vi "3.1.0_ECO_Mode.vi"(6 "Data in":T2, 8 "error in (no error)":errorcluster, 9 "AllControls In":T1, 10 "?":T3, 11 "Message Queue out":T4) -> (0 "error out":errorcluster, 1 "Flow":string, 2 "Data":T3, 3 "Message Queue Out":T4, 4 "Data out":T2)   [LabVIEW 2017]
uses:
  Depends/AMC/subVIs/TypeDefs/amc_Message Queue.ctl
  Depends/AMC/subVIs/TypeDefs/amc_Message.ctl
  Depends/Tools/Keyed Array/Tools_KeyedArray KeyedArray.ctl
  Ctrls/Data.ctl
  Ctrls/CSV_Data.ctl
  Ctrls/AllControls.ctl
  Ctrls/AlarmIndex.ctl
  DIPC 692 Daemon API/typdef/get_parameter.ctl
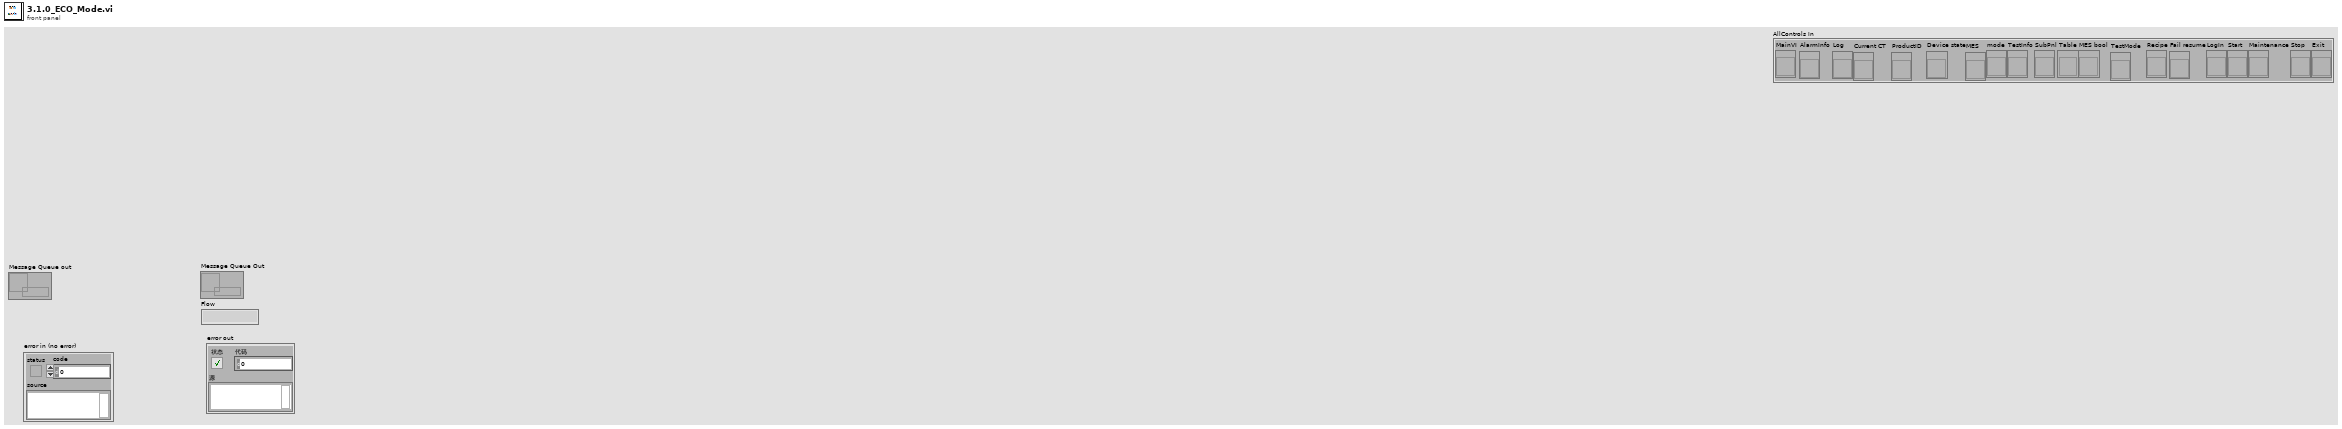
[diagram p1: front panel]
types:
  T1 = typedef "AllControls.ctl" = cluster{"MainVI":refnum<vi>, "AlarmInfo":refnum<vi>, "Log":refnum<vi>, "Current CT":refnum<vi>, "ProductID":refnum<vi>, "Device state":refnum<vi>, "MES":refnum<vi>, "mode":refnum<vi>, "TestInfo":refnum<vi>, "SubPnl":refnum<vi>, "Table":refnum<vi>, "MES bool":refnum<vi>, "TestMode":refnum<vi>, "Recipe":refnum<vi>, "Fail resume":refnum<vi>, "LogIn":refnum<vi>, "Start":refnum<vi>, "Maintenance":refnum<vi>, "Stop":refnum<vi>, "Exit":refnum<vi>}
  T2 = typedef "CSV_Data.ctl" = cluster{"Initialisation":cluster{"LMT - Connect UUT (con COM)":string, "LMT - Software Version (rrel)":string, "LMT - Write SKU file (wskuc)":string, "LMT - SKU file name":string, "Connect UUT DDM":string, "Read DDM EOL Timestamp - Mode":string, "Read DDM EOL Timestamp - Timestamp":string, "Read DDM EOL Timestamp - Rig ID":string, "Read DDM EOL Timestamp - Passmark ID":string, "Read DDM EOL Timestamp - Passmark Rev":string, "Software Version before flashing":string, "Read Hardware Serial":string, "UUT DDM SN":string, "Compare DDM SN with MES SN":string, "Backup PCBA Calibration EEPROM Response - CAL":string, "Flash Firmware Version":string, "Check SW Version":string, "Read DDM SW Version after flashing":string, "Set SKU Config":string, "Ready Status":string, "Set Device Mode to EOL":string, "DDM Parameter - Voltage":string, "DDM Parameter - Current":string, "DDM Parameter - Power":string, "DDM Parameter - Speed":string, "DDM Parameter - Pressure":string, "Tester Parameter - Voltage":string, "Tester Parameter - Current":string, "Tester Parameter - Power":string, "Tester Parameter - Ambient Pressure":string, "Tester Parameter - Ambient Temperature":string, "Calculated Parameter - DDM Pressure Corrected":string, "Calculated Parameter - DDM Real Power":string, "Calculated Parameter - Delta V":string}, "BEMF_Calibration":cluster{"Calibration Result - eol_cold_bemf_temp":string, "DDM Ambient Temp":string, "Restriction Plate Diameter":string, "Calibration Result - eol_bemf_mp_cold_coef_a":string, "Calibration Result - eol_bemf_mp_cold_coef_b":string, "Calibration Result - eol_bemf_mp_cold_coef_c":string, "Calibration Result - eol_bemf_lsi_cold_ref_coeffs":string, "Get - Calibration Result - eol_bemf_lsi_speed":string, "Get - Calibration Result - eol_bemf_lsi_integral_0":string, "Calibration Result - eol_bemf_lsi_integral_1":string, "Get - Calibration Result - eol_bemf_lsi_integral_2":string, "Get - Calibration Result - eol_cold_bemf":string, "Get - Calibration Result - eol_cold_bemf_fisf":string, "Finalise Calibration":string, "Compare -Calibration Result - eol_cold_bemf":string, "Compare -Calibration Result - eol_cold_bemf_fisf":string}, "ECO":cluster{"Reset Power Tune":string, "Reset BEMF FISF Calibration":string, "Restriction Plate Diameter":string, "ECO - Stabilisation Time":string, "ECO - DDM Parameter - Voltage":string, "ECO - DDM Parameter - Current":string, "ECO - DDM Parameter - Power":string, "ECO - DDM Parameter - Measured Power":string, "ECO - DDM Parameter - Speed":string, "ECO - DDM Parameter - Pressure":string, "ECO - Tester Parameter - Voltage":string, "ECO - Tester Parameter - Current":string, "ECO - Tester Parameter - Power":string, "ECO - Tester Parameter - Ambient Pressure":string, "ECO - Tester Parameter - Ambient Temperature":string, "ECO - Tester Parameter - Ambient Humidity":string, "ECO - Calculated Parameter - DDM Pressure Corrected":string, "ECO - Calculated Parameter - DDM Real Power":string, "ECO - Calculated Parameter - Delta V":string, "ECO - Calculated Parameter - Flowrate":string, "ECO - Calculated Parameter - Airwatt":string, "ECO - Formula":string, "PT ECO - Power Tune Mode Status":string}, "BOOST":cluster{"Restriction Plate Diameter":string, "BOOST - Stabilisation Time":string, "BOOST - DDM Parameter - Voltage":string, "BOOST - DDM Parameter - Current":string, "BOOST - DDM Parameter - Power":string, "BOOST - DDM Parameter - Measured Power":string, "BOOST - DDM Parameter - Speed":string, "BOOST - DDM Parameter - Pressure":string, "BOOST - Tester Parameter - Voltage":string, "BOOST - Tester Parameter - Current":string, "BOOST - Tester Parameter - Power":string, "BOOST - Tester Parameter - Ambient Pressure":string, "BOOST - Tester Parameter - Ambient Temperature":string, "BOOST - Tester Parameter - Ambient Humidity":string, "BOOST - Calculated Parameter - DDM Pressure Corrected":string, "BOOST - Calculated Parameter - DDM Real Power":string, "BOOST - Calculated Parameter - Delta V":string, "BOOST - Calculated Parameter - Flowrate":string, "BOOST - Calculated Parameter - Airwatt":string, "BOOST - Get AM Presence":string, "Air Muscle Turn Off Status":string, "BOOST - Air Muscle Calculated Parameter - Airwatt B":string, "BOOST - Air Muscle Calculate Airwatt Delta":string, "PT BOOST - Power Tune Mode Status":string, "Finalise Calibration":string, "ECO - Get AW Calibration value":string, "BOOST - Get AW Calibration value":string}, "MAX":cluster{"Restriction Plate Diameter":string, "MAX - Stabilisation Time":string, "Get Average Delta Tmag (LSIdelta_FISFdelta_LSItmag_FISFtmag_IIRtmag)":string, "Get Average Delta Tmag FISF":string, "MAX - DDM Parameter - Voltage":string, "MAX - DDM Parameter - Current":string, "MAX - DDM Parameter - Power":string, "MAX - DDM Parameter - Measured Power":string, "MAX - DDM Parameter - Speed":string, "MAX - DDM Parameter - Pressure":string, "MAX - Tester Parameter - Voltage":string, "MAX - Tester Parameter - Current":string, "MAX - Tester Parameter - Power":string, "MAX - Tester Parameter - Ambient Pressure":string, "MAX - Tester Parameter - Ambient Temperature":string, "MAX - Tester Parameter - Ambient Humidity":string, "MAX - Calculated Parameter - DDM Pressure Corrected":string, "MAX - Calculated Parameter - DDM Real Power":string, "MAX - Calculated Parameter - Delta V":string, "MAX - Calculated Parameter - Flowrate":string, "MAX - Calculated Parameter - Airwatt":string, "MAX_FISF_Check_Average_Delta_Tmag":string, "MAX - FISF - BEMF Finetune Result":string, "MAX tune - Delta P1":string, "MAX tune - Calculated Parameter - Airwatt":string, "Calculate Delta Airwatts - MAX finetune - Delta P2":string, "MAX finetune - DDM Parameter - Voltage":string, "MAX finetune - DDM Parameter - Current":string, "MAX finetune - DDM Parameter - Power":string, "MAX finetune - DDM Parameter - Measured Power":string, "MAX finetune - DDM Parameter - Speed":string, "MAX finetune - DDM Parameter - Pressure":string, "MAX finetune - Tester Parameter - Voltage":string, "MAX finetune - Tester Parameter - Current":string, "MAX finetune - Tester Parameter - Power":string, "MAX finetune - Tester Parameter - Ambient Pressure":string, "MAX finetune - Tester Parameter - Ambient Temperature":string, "MAX finetune - Tester Parameter - Ambient Humidity":string, "MAX finetune - Calculated Parameter - DDM Pressure Corrected":string, "MAX finetune - Calculated Parameter - DDM Real Power":string, "MAX finetune - Calculated Parameter - Delta V":string, "MAX finetune - Calculated Parameter - Flowrate":string, "MAX finetune - Calculated Parameter - Airwatt":string, "Check Derate Result":string, "Delta Tmag FISF":string, "Get Hot BEMF Result":string, "Calculate delta Pressure":string, "Finalise Calibration":string, "Calculate & Check Delta BEMF":string, "Delta P Airwatts Value":string}, "LL":cluster{"DDM Ambient Temp":string, "Restriction Plate Diameter":string, "LL - DDM Parameter - Voltage":string, "LL - DDM Parameter - Current":string, "LL - DDM Parameter - Power":string, "LL - DDM Parameter - Measured Power":string, "LL - DDM Parameter - Speed":string, "LL - DDM Parameter - Pressure":string, "LL - Tester Parameter - Voltage":string, "LL - Tester Parameter - Current":string, "LL - Tester Parameter - Power":string, "LL - DDM Real Power":string, "LL - Calibrate Task Detect LL":string}, "HL":cluster{"HL - DDM Parameter - Voltage":string, "HL - DDM Parameter - Current":string, "HL - DDM Parameter - Power":string, "HL - DDM Parameter - Measured Power":string, "HL - DDM Parameter - Speed":string, "HL - DDM Parameter - Pressure":string, "HL - Tester Parameter - Voltage":string, "HL - Tester Parameter - Current":string, "HL - Tester Parameter - Power":string, "HL - DDM Real Power":string, "HL - Calibrate Task Detect HL":string}, "LH":cluster{"Restriction Plate Diameter":string, "LH - DDM Parameter - Voltage":string, "LH - DDM Parameter - Current":string, "LH - DDM Parameter - Power":string, "LH - DDM Parameter - Measured Power":string, "LH - DDM Parameter - Speed":string, "LH - DDM Parameter - Pressure":string, "LH - Tester Parameter - Voltage":string, "LH - Tester Parameter - Current":string, "LH - Tester Parameter - Power":string, "LH - DDM Real Power":string, "LH - Calibrate Task Detect LH":string}, "HH":cluster{"HH - DDM Parameter - Voltage":string, "HH - DDM Parameter - Current":string, "HH - DDM Parameter - Power":string, "HH - DDM Parameter - Measured Power":string, "HH - DDM Parameter - Speed":string, "HH - DDM Parameter - Pressure":string, "HH - Tester Parameter - Voltage":string, "HH - Tester Parameter - Current":string, "HH - Tester Parameter - Power":string, "HH - DDM Real Power":string, "HH - Calibrate Task Detect HH":string}, "Inlet Blockage Calibration":cluster{"Inlet Blockage Calibration - DDM Parameter - Voltage":string, "Inlet Blockage Calibration - DDM Parameter - Current":string, "Inlet Blockage Calibration - DDM Parameter - Power":string, "Inlet Blockage Calibration - DDM Parameter - Measured Power":string, "Inlet Blockage Calibration - DDM Parameter - Speed":string, "Inlet Blockage Calibration - DDM Parameter - Pressure":string, "Inlet Blockage Calibration - Tester Parameter - Voltage":string, "Inlet Blockage Calibration - Tester Parameter - Current":string, "Inlet Blockage Calibration - Tester Parameter - Power":string, "Inlet Blockage Calibration - DDM Real Power":string, "Calibration Inlet Blockage_E":string, "Finalise Calibration":string, "Get Task Detect LL":string, "Get Task Detect HL":string, "Get Task Detect LH":string, "Get Task Detect HH":string, "Calibration Inlet Blockage":string, "Calibration eol cold bemf temp":string}, "GOOD":cluster{"GOOD UNIT - Clear EEPROM Error Log":string, "GOOD UNIT - Write Product Timestamp - Mode":string, "GOOD UNIT - Write Product Timestamp - Timestamp":string, "GOOD UNIT - Write Product Timestamp - Rig ID":string, "GOOD UNIT - Write Product Timestamp - Passmark ID":string, "GOOD UNIT - Write Product Timestamp - Passmark Rev":string, "GOOD UNIT - Set Device Mode to PROD":string, "GOOD UNIT - Backup PCBA Calibration EEPROM Response":string, "GOOD UNIT - Check Security Bit":string, "GOOD UNIT - Set Calibration Lock":string, "GOOD UNIT - Get_Calibration_Lock":string, "GOOD UNIT - Disconnect UUT":string}, "NG":cluster{"NG UNIT - Read NVM Error":string, "NG UNIT - Set Device Mode to FCT":string, "NG UNIT - Backup PCBA Calibration EEPROM Response - CAL":string, "NG UNIT - Backup PCBA Calibration EEPROM Response - ERROR":string, "NG UNIT - Backup PCBA Calibration EEPROM Response - USAGE":string, "NG UNIT - Disconnect UUT":string}, "SN":string, "Table":string[][], "Count":cluster{"Total":i32, "OK":i32, "NG":i32, "Yield":dbl}, "Start Time":timestamp, "daemon reference":refnum<k5>, "CT":dbl, "Config":string[][], "OK/NG":bool, "Station ID":string, "MES DDM SN":string, "MES PCBA SN":string, "Retest":string, "Variant":string, "Initialisation_Status":cluster{"LMT - Connect UUT (con COM)":string, "LMT - Software Version (rrel)":string, "LMT - Write SKU file (wskuc)":string, "LMT - SKU file name":string, "Connect UUT DDM":string, "Read DDM EOL Timestamp - Mode":string, "Read DDM EOL Timestamp - Timestamp":string, "Read DDM EOL Timestamp - Rig ID":string, "Read DDM EOL Timestamp - Passmark ID":string, "Read DDM EOL Timestamp - Passmark Rev":string, "Software Version before flashing":string, "Read Hardware Serial":string, "UUT DDM SN":string, "Compare DDM SN with MES SN":string, "Backup PCBA Calibration EEPROM Response - CAL":string, "Flash Firmware Version":string, "Check SW Version":string, "Read DDM SW Version after flashing":string, "Set SKU Config":string, "Ready Status":string, "Set Device Mode to EOL":string, "DDM Parameter - Voltage":string, "DDM Parameter - Current":string, "DDM Parameter - Power":string, "DDM Parameter - Speed":string, "DDM Parameter - Pressure":string, "Tester Parameter - Voltage":string, "Tester Parameter - Current":string, "Tester Parameter - Power":string, "Tester Parameter - Ambient Pressure":string, "Tester Parameter - Ambient Temperature":string, "Calculated Parameter - DDM Pressure Corrected":string, "Calculated Parameter - DDM Real Power":string, "Calculated Parameter - Delta V":string}, "BEMF_Calibration_Status":cluster{"Calibration Result - eol_cold_bemf_temp":string, "DDM Ambient Temp":string, "Restriction Plate Diameter":string, "Calibration Result - eol_bemf_mp_cold_coef_a":string, "Calibration Result - eol_bemf_mp_cold_coef_b":string, "Calibration Result - eol_bemf_mp_cold_coef_c":string, "Calibration Result - eol_bemf_lsi_cold_ref_coeffs":string, "Get - Calibration Result - eol_bemf_lsi_speed":string, "Get - Calibration Result - eol_bemf_lsi_integral_0":string, "Calibration Result - eol_bemf_lsi_integral_1":string, "Get - Calibration Result - eol_bemf_lsi_integral_2":string, "Get - Calibration Result - eol_cold_bemf":string, "Get - Calibration Result - eol_cold_bemf_fisf":string, "Finalise Calibration":string, "Compare -Calibration Result - eol_cold_bemf":string, "Compare -Calibration Result - eol_cold_bemf_fisf":string}, "ECO_Status":cluster{"Reset Power Tune":string, "Reset BEMF FISF Calibration":string, "Restriction Plate Diameter":string, "ECO - Stabilisation Time":string, "ECO - DDM Parameter - Voltage":string, "ECO - DDM Parameter - Current":string, "ECO - DDM Parameter - Power":string, "ECO - DDM Parameter - Measured Power":string, "ECO - DDM Parameter - Speed":string, "ECO - DDM Parameter - Pressure":string, "ECO - Tester Parameter - Voltage":string, "ECO - Tester Parameter - Current":string, "ECO - Tester Parameter - Power":string, "ECO - Tester Parameter - Ambient Pressure":string, "ECO - Tester Parameter - Ambient Temperature":string, "ECO - Tester Parameter - Ambient Humidity":string, "ECO - Calculated Parameter - DDM Pressure Corrected":string, "ECO - Calculated Parameter - DDM Real Power":string, "ECO - Calculated Parameter - Delta V":string, "ECO - Calculated Parameter - Flowrate":string, "ECO - Calculated Parameter - Airwatt":string, "ECO - Formula":string, "PT ECO - Power Tune Mode Status":string}, "BOOST_Status":cluster{"Restriction Plate Diameter":string, "BOOST - Stabilisation Time":string, "BOOST - DDM Parameter - Voltage":string, "BOOST - DDM Parameter - Current":string, "BOOST - DDM Parameter - Power":string, "BOOST - DDM Parameter - Measured Power":string, "BOOST - DDM Parameter - Speed":string, "BOOST - DDM Parameter - Pressure":string, "BOOST - Tester Parameter - Voltage":string, "BOOST - Tester Parameter - Current":string, "BOOST - Tester Parameter - Power":string, "BOOST - Tester Parameter - Ambient Pressure":string, "BOOST - Tester Parameter - Ambient Temperature":string, "BOOST - Tester Parameter - Ambient Humidity":string, "BOOST - Calculated Parameter - DDM Pressure Corrected":string, "BOOST - Calculated Parameter - DDM Real Power":string, "BOOST - Calculated Parameter - Delta V":string, "BOOST - Calculated Parameter - Flowrate":string, "BOOST - Calculated Parameter - Airwatt":string, "BOOST - Get AM Presence":string, "Air Muscle Turn Off Status":string, "BOOST - Air Muscle Calculated Parameter - Airwatt B":string, "BOOST - Air Muscle Calculate Airwatt Delta":string, "PT BOOST - Power Tune Mode Status":string, "Finalise Calibration":string, "ECO - Get AW Calibration value":string, "BOOST - Get AW Calibration value":string}, "MAX_Status":cluster{"Restriction Plate Diameter":string, "MAX - Stabilisation Time":string, "Get Average Delta Tmag (LSIdelta_FISFdelta_LSItmag_FISFtmag_IIRtmag)":string, "Get Average Delta Tmag FISF":string, "MAX - DDM Parameter - Voltage":string, "MAX - DDM Parameter - Current":string, "MAX - DDM Parameter - Power":string, "MAX - DDM Parameter - Measured Power":string, "MAX - DDM Parameter - Speed":string, "MAX - DDM Parameter - Pressure":string, "MAX - Tester Parameter - Voltage":string, "MAX - Tester Parameter - Current":string, "MAX - Tester Parameter - Power":string, "MAX - Tester Parameter - Ambient Pressure":string, "MAX - Tester Parameter - Ambient Temperature":string, "MAX - Tester Parameter - Ambient Humidity":string, "MAX - Calculated Parameter - DDM Pressure Corrected":string, "MAX - Calculated Parameter - DDM Real Power":string, "MAX - Calculated Parameter - Delta V":string, "MAX - Calculated Parameter - Flowrate":string, "MAX - Calculated Parameter - Airwatt":string, "MAX_FISF_Check_Average_Delta_Tmag":string, "MAX - FISF - BEMF Finetune Result":string, "MAX tune - Delta P1":string, "MAX tune - Calculated Parameter - Airwatt":string, "Calculate Delta Airwatts - MAX finetune - Delta P2":string, "MAX finetune - DDM Parameter - Voltage":string, "MAX finetune - DDM Parameter - Current":string, "MAX finetune - DDM Parameter - Power":string, "MAX finetune - DDM Parameter - Measured Power":string, "MAX finetune - DDM Parameter - Speed":string, "MAX finetune - DDM Parameter - Pressure":string, "MAX finetune - Tester Parameter - Voltage":string, "MAX finetune - Tester Parameter - Current":string, "MAX finetune - Tester Parameter - Power":string, "MAX finetune - Tester Parameter - Ambient Pressure":string, "MAX finetune - Tester Parameter - Ambient Temperature":string, "MAX finetune - Tester Parameter - Ambient Humidity":string, "MAX finetune - Calculated Parameter - DDM Pressure Corrected":string, "MAX finetune - Calculated Parameter - DDM Real Power":string, "MAX finetune - Calculated Parameter - Delta V":string, "MAX finetune - Calculated Parameter - Flowrate":string, "MAX finetune - Calculated Parameter - Airwatt":string, "Check Derate Result":string, "Delta Tmag FISF":string, "Get Hot BEMF Result":string, "Calculate delta Pressure":string, "Finalise Calibration":string, "Calculate & Check Delta BEMF":string, "Delta P Airwatts Value":string}, "LL_Status":cluster{"DDM Ambient Temp":string, "Restriction Plate Diameter":string, "LL - DDM Parameter - Voltage":string, "LL - DDM Parameter - Current":string, "LL - DDM Parameter - Power":string, "LL - DDM Parameter - Measured Power":string, "LL - DDM Parameter - Speed":string, "LL - DDM Parameter - Pressure":string, "LL - Tester Parameter - Voltage":string, "LL - Tester Parameter - Current":string, "LL - Tester Parameter - Power":string, "LL - DDM Real Power":string, "LL - Calibrate Task Detect LL":string}, "HL_Status":cluster{"HL - DDM Parameter - Voltage":string, "HL - DDM Parameter - Current":string, "HL - DDM Parameter - Power":string, "HL - DDM Parameter - Measured Power":string, "HL - DDM Parameter - Speed":string, "HL - DDM Parameter - Pressure":string, "HL - Tester Parameter - Voltage":string, "HL - Tester Parameter - Current":string, "HL - Tester Parameter - Power":string, "HL - DDM Real Power":string, "HL - Calibrate Task Detect HL":string}, "LH_Status":cluster{"Restriction Plate Diameter":string, "LH - DDM Parameter - Voltage":string, "LH - DDM Parameter - Current":string, "LH - DDM Parameter - Power":string, "LH - DDM Parameter - Measured Power":string, "LH - DDM Parameter - Speed":string, "LH - DDM Parameter - Pressure":string, "LH - Tester Parameter - Voltage":string, "LH - Tester Parameter - Current":string, "LH - Tester Parameter - Power":string, "LH - DDM Real Power":string, "LH - Calibrate Task Detect LH":string}, "HH_Status":cluster{"HH - DDM Parameter - Voltage":string, "HH - DDM Parameter - Current":string, "HH - DDM Parameter - Power":string, "HH - DDM Parameter - Measured Power":string, "HH - DDM Parameter - Speed":string, "HH - DDM Parameter - Pressure":string, "HH - Tester Parameter - Voltage":string, "HH - Tester Parameter - Current":string, "HH - Tester Parameter - Power":string, "HH - DDM Real Power":string, "HH - Calibrate Task Detect HH":string}, "Inlet Blockage Calibration_Status":cluster{"Inlet Blockage Calibration - DDM Parameter - Voltage":string, "Inlet Blockage Calibration - DDM Parameter - Current":string, "Inlet Blockage Calibration - DDM Parameter - Power":string, "Inlet Blockage Calibration - DDM Parameter - Measured Power":string, "Inlet Blockage Calibration - DDM Parameter - Speed":string, "Inlet Blockage Calibration - DDM Parameter - Pressure":string, "Inlet Blockage Calibration - Tester Parameter - Voltage":string, "Inlet Blockage Calibration - Tester Parameter - Current":string, "Inlet Blockage Calibration - Tester Parameter - Power":string, "Inlet Blockage Calibration - DDM Real Power":string, "Calibration Inlet Blockage_E":string, "Finalise Calibration":string, "Get Task Detect LL":string, "Get Task Detect HL":string, "Get Task Detect LH":string, "Get Task Detect HH":string, "Calibration Inlet Blockage":string, "Calibration eol cold bemf temp":string}, "GOOD_Status":cluster{"GOOD UNIT - Clear EEPROM Error Log":string, "GOOD UNIT - Write Product Timestamp - Mode":string, "GOOD UNIT - Write Product Timestamp - Timestamp":string, "GOOD UNIT - Write Product Timestamp - Rig ID":string, "GOOD UNIT - Write Product Timestamp - Passmark ID":string, "GOOD UNIT - Write Product Timestamp - Passmark Rev":string, "GOOD UNIT - Set Device Mode to PROD":string, "GOOD UNIT - Backup PCBA Calibration EEPROM Response":string, "GOOD UNIT - Check Security Bit":string, "GOOD UNIT - Set Calibration Lock":string, "GOOD UNIT - Get_Calibration_Lock":string, "GOOD UNIT - Disconnect UUT":string}, "NG_Status":cluster{"NG UNIT - Read NVM Error":string, "NG UNIT - Set Device Mode to FCT":string, "NG UNIT - Backup PCBA Calibration EEPROM Response - CAL":string, "NG UNIT - Backup PCBA Calibration EEPROM Response - ERROR":string, "NG UNIT - Backup PCBA Calibration EEPROM Response - USAGE":string, "NG UNIT - Disconnect UUT":string}, "SKU":string, "Plate_Diameter":string, "Alarm":string}
  T3 = typedef "Data.ctl" = cluster{"Initialisation":cluster{"DDM_Parameter":dbl[], "DDM_Parameter_status":bool[], "Get_Tester_Parameter":dbl[], "Get_Tester_Parameter_status":bool[], "Cal_Tester_Parameter":dbl[], "Cal_Tester_Parameter_status":bool[], "sw_version_before_status":bool, "sw_version_after_status":bool, "Set_SKU_Config_With_LMT_status":bool, "FCT_timestamp_status":bool, "LMT_Connect_to_UUT_status":bool}, "BEMF_Calibration":cluster{"Read_ambient_temperature":dbl, "Calibration_Vaule":dbl[], "Calibration_Vaule _B":dbl[], "Calibration_Vaule_status":bool[], "Calibration_Vaule_B_status":bool[]}, "ECO":cluster{"DDM_Parameter":dbl[], "DDM_Parameter_status":bool[], "Get_Tester_Parameter":dbl[], "Get_Tester_Parameter_status":bool[], "Cal_Tester_Parameter":dbl[], "Cal_Tester_Parameter_status":bool[], "DDM_Parameter_after_power_tune":dbl[], "Get_Tester_Parameter_after_power_tune":dbl[], "Cal_Tester_Parameter_after_power_tune":dbl[], "Cal_Tester_Parameter_after_power_tune_status":bool[], "Delta_P":dbl}, "BOOST":cluster{"DDM_Parameter":dbl[], "DDM_Parameter_status":bool[], "Get_Tester_Parameter":dbl[], "Get_Tester_Parameter_status":bool[], "Cal_Tester_Parameter":dbl[], "Cal_Tester_Parameter_status":bool[], "DDM_Parameter_after_power_tune":dbl[], "Get_Tester_Parameter_after_power_tune":dbl[], "Cal_Tester_Parameter_after_power_tune":dbl[], "Cal_Tester_Parameter_after_power_tune_status":bool[], "airwatts_am_off":dbl, "AW_Delta_(AM_on_and_off)":dbl, "AW_Delta_(AM_on_and_off)_Status":bool, "Delta_P":dbl}, "MAX":cluster{"Average_Tmag_Data":cluster{"LSI Delta in degC":dbl, "FISF Delta in degc":dbl, "LSI Tmag in degC":dbl, "Fisf Tmag in degC":dbl, "IIR Tmag in degC":dbl}, "DDM_Parameter":dbl[], "DDM_Parameter_status":bool[], "Get_Tester_Parameter":dbl[], "Get_Tester_Parameter_status":bool[], "Cal_Tester_Parameter":dbl[], "BEMF_Finetune":cluster{"eol_bemf_mp_cold_coef_c":dbl, "eol_cold_bemf_fisf_offset":dbl}, "AW_Tune":cluster{"delta_P1":dbl, "delta_P_Setting":dbl}, "DDM_Parameter_after_Airwatts_Tune":dbl[], "Get_Tester_Parameter_after_Airwatts_Tune":dbl[], "Cal_Tester_Parameter_after_Airwatts_Tune":dbl[], "DDM_Parameter_after_Airwatts_Finetune":dbl[], "Get_Tester_Parameter_after_Airwatts_Finetune":dbl[], "Cal_Tester_Parameter_after_Airwatts_Finetune":dbl[], "AW_Finetune":cluster{"delta_P2":dbl, "delta_P_Setting":dbl}, "Delta_Tmag_after_tune":cluster{"LSI Delta in degC":dbl, "FISF Delta in degc":dbl, "LSI Tmag in degC":dbl, "Fisf Tmag in degC":dbl, "IIR Tmag in degC":dbl}, "Hot Bemf in mV":dbl, "DDM_Pressure":dbl, "Delta_Pressure":dbl, " Cold Bemf in mV":dbl, " delta Bemf":dbl, " delta p":dbl, "Delta_Pressure_status":bool, " delta Bemf_status":bool, "LSI Delta in degC_status":bool, "FISF Delta in degc_status":bool, "Max_check_derate_status_status":bool, "Average_All_data":dbl[][], "Average_Tmag_Data_status":bool[], "Average_Tmag_Data_after_tune_status":bool[], "Cal_Tester_Parameter_status":bool[], "Cal_Tester_Parameter_status_after_Airwatts_Tune":bool[], "Cal_Tester_Parameter_status_after_Airwatts_FineTune":bool[]}, "Task_Detect_Calib":cluster{"LL":cluster{"DDM_Parameter":dbl[], "DDM_Parameter_status":bool[], "Get_Tester_Parameter":dbl[], "Get_Tester_Parameter_status":bool[], "Set_task_detect_A":dbl, "Set_task_detect_A_Status":bool}, "HL":cluster{"DDM_Parameter":dbl[], "DDM_Parameter_status":bool[], "Get_Tester_Parameter":dbl[], "Get_Tester_Parameter_status":bool[], "Set_task_detect_B":dbl, "Set_task_detect_B_Status":bool}, "LH":cluster{"DDM_Parameter":dbl[], "DDM_Parameter_status":bool[], "Get_Tester_Parameter":dbl[], "Get_Tester_Parameter_status":bool[], "Set_task_detect_C":dbl, "Set_task_detect_C_Status":bool}, "HH":cluster{"DDM_Parameter":dbl[], "DDM_Parameter_status":bool[], "Get_Tester_Parameter":dbl[], "Get_Tester_Parameter_status":bool[], "Set_task_detect_D":dbl, "Read_and_check_calibration_Status":bool[], "Set_task_detect_D_Status":bool}, "Get_eol_inlet_blockage_E":dbl, "Calib_vaule":cluster{"Get_task_detect_LL":dbl, "Get_task_detect_HL":dbl, "Get_task_detect_LH":dbl, "Get_task_detect_HH":dbl, "eol_inlet_blockage":dbl, "eol_code_bemf_temp":dbl}, "calibrated temp":dbl, "Inlet_Blockage_Calibration":cluster{"DDM_Parameter":dbl[], "DDM_Parameter_status":bool[], "Get_Tester_Parameter":dbl[], "Get_Tester_Parameter_status":bool[]}, "Get_eol_inlet_blockage_E_Status":bool}, "good":cluster{"Write_Product_TS":cluster{"TIMESTAMP":i64, "RIG_ID":i64, "PASSMARK_ID":i64, "PASSMARK_REV":i64}, "Read_Product_TS":cluster{"TIMESTAMP":i64, "RIG_ID":i64, "PASSMARK_ID":i64, "PASSMARK_REV":i64}, "Good_Check_Secuity_Bit_Stauts":bool}}
  T4 = typedef "amc_Message Queue.ctl" = refnum<queue>
  T5 = typedef "HD Config.ctl" = cluster{" PC":cluster{"PC Address":u8[], "PC Port":i32}, "FCO":cluster{"COM":refnum<visa-resource-name>, "Baudrate":u32}, "DC Power ":cluster{"COM":refnum<visa-resource-name>, "Baudrate":u32}, "PW3336":cluster{"COM":refnum<visa-resource-name>, "Baudrate":u32}, "Lefoo":cluster{"COM":refnum<visa-resource-name>, "Baudrate":u32}, "AI Model":cluster{"COM":refnum<visa-resource-name>, "Baudrate":u32}, "DIPC":cluster{"COM":refnum<visa-resource-name>}, "NFC":cluster{"IP Address":string, "Port":u16, "Retry":u16}, "Motor":cluster{"COM":refnum<visa-resource-name>, "Baudrate":u32}, "Fail_resume_mode":bool, "GRR":bool}
  T6 = typedef "AlarmIndex.ctl" = enum16{"E-Stop", "Safety light grid", "UUT Sealing Cylinder HomePoint", "UUT Sealing Cylinder WorkPoint", "Orifice fixed Cylinder L HomePoint", "Orifice fixed Cylinder L WorkPoint", "Orifice fixed Cylinder R HomePoint", "Orifice fixed Cylinder R WorkPoint", "UUT Cylinder HomePoint", "UUT Cylinder WorkPoint", "Carrier fixed Cylinder L HomePoint", "Carrier fixed Cylinder L WorkPoint", "Carrier fixed Cylinder R HomePoint", "Carrier fixed Cylinder R WorkPoint", "Probe Cylinder HomePoint", "Probe Cylinder WorkPoint", "Motor Error", "Test Error"}
  T7 = typedef "get_parameter.ctl" = string
  T8 = typedef "Position Config.ctl" = cluster{"OrificeSize_12.7":i32, "OrificeSize_13":i32, "OrificeSize_30":i32, "OrificeSize_16":i32}
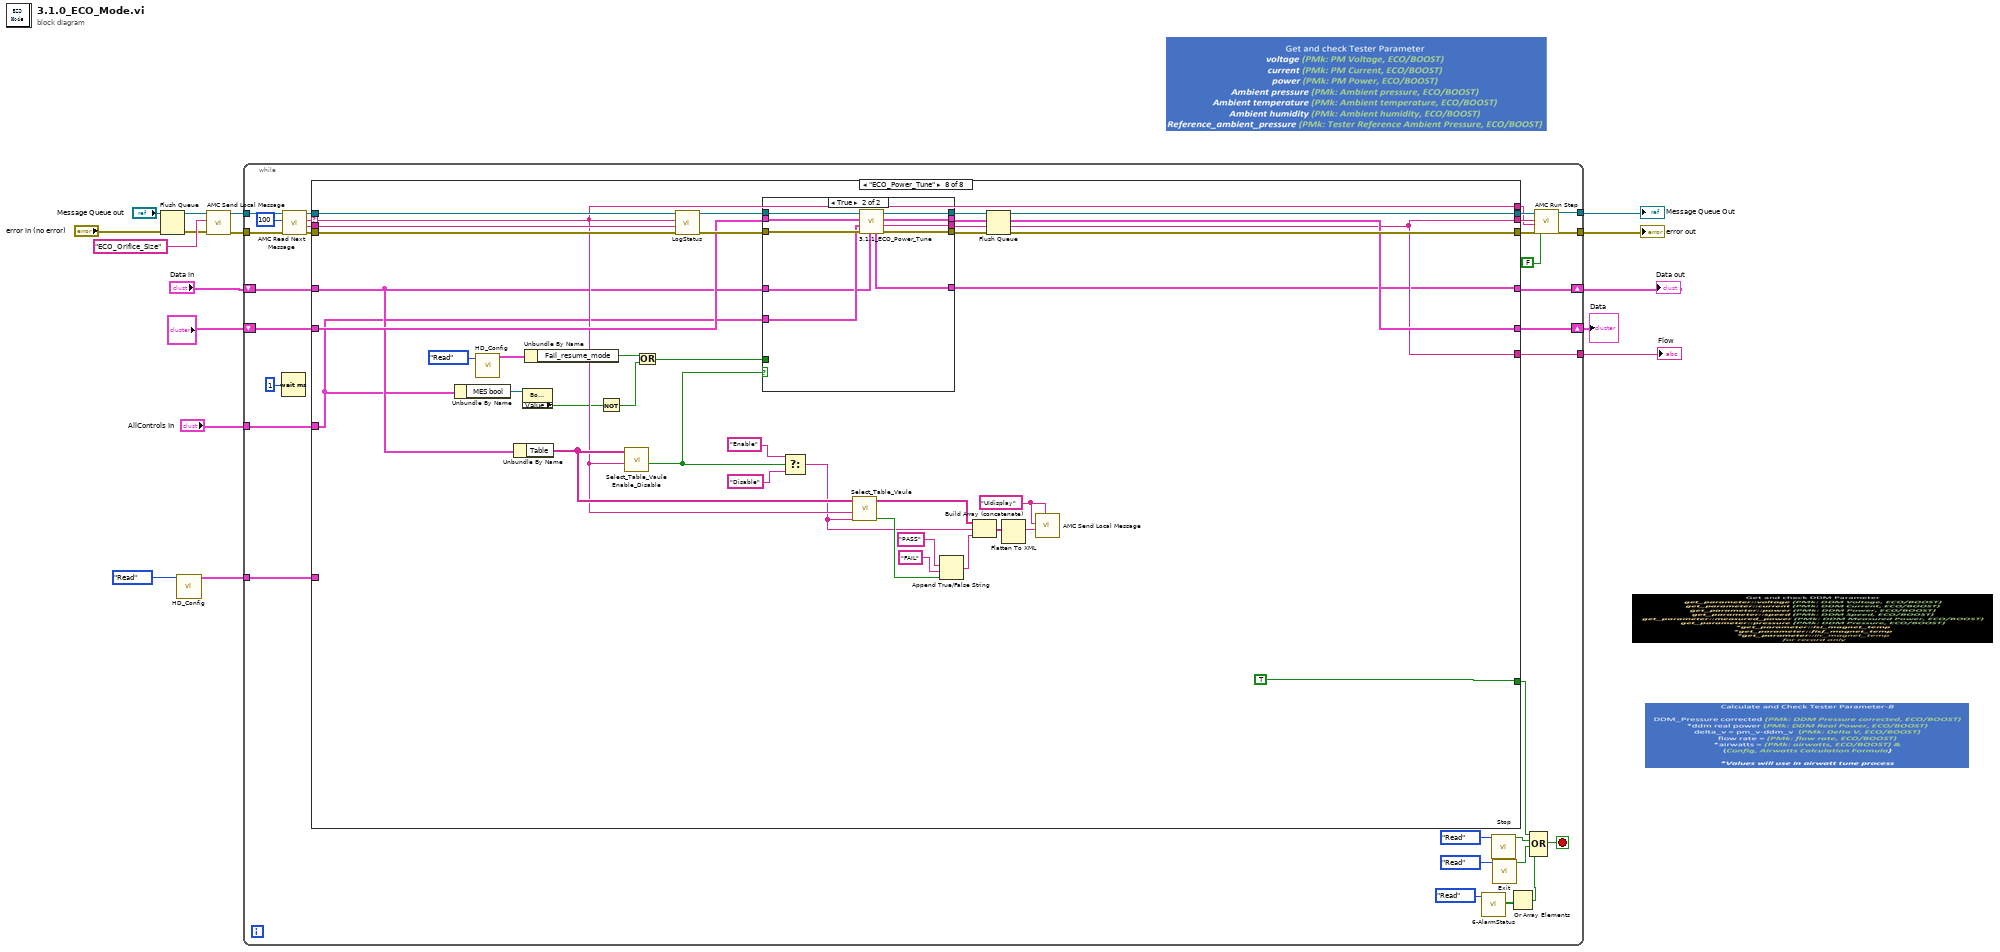
[diagram p0: block diagram]
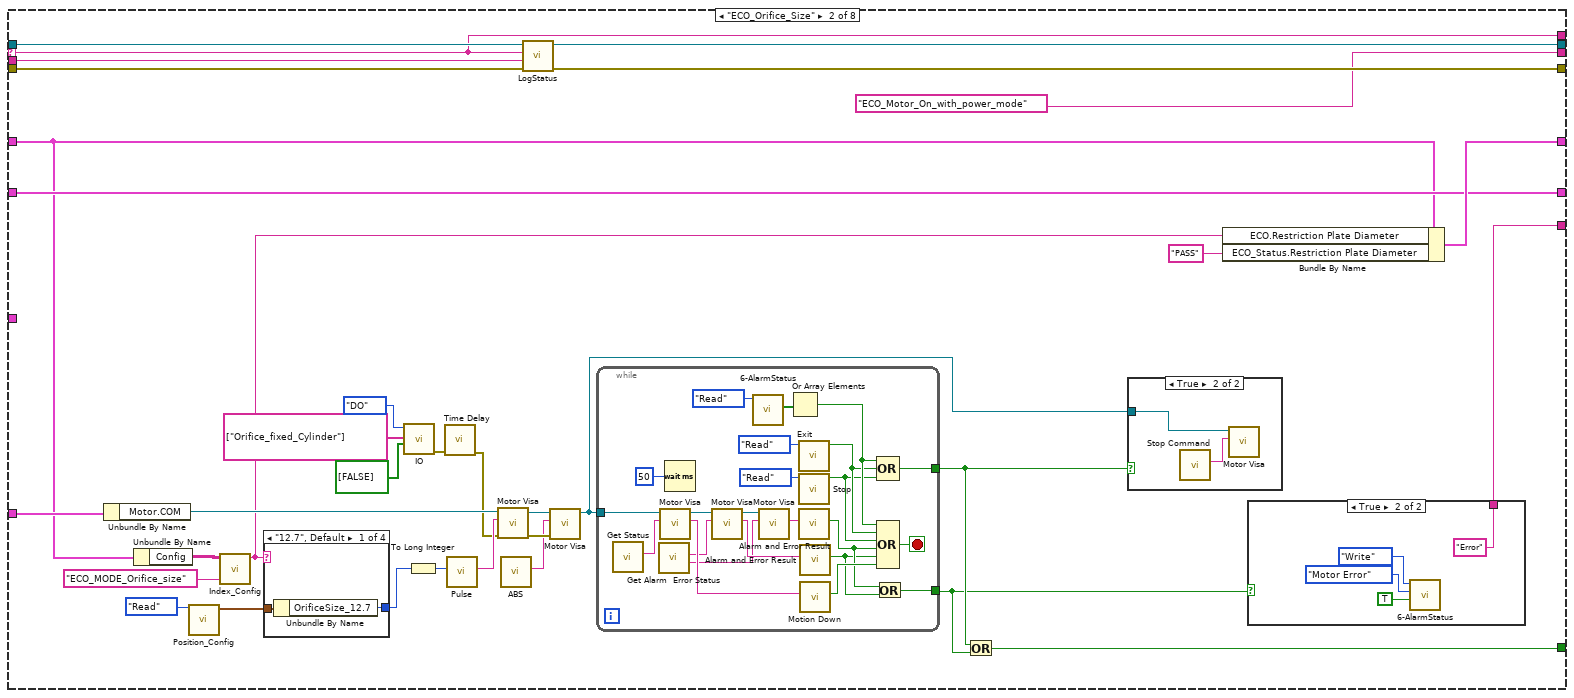
[diagram p3: hidden frame]
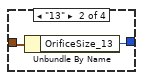
[diagram p5: hidden frame]
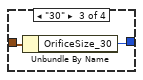
[diagram p6: hidden frame]
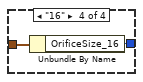
[diagram p7: hidden frame]
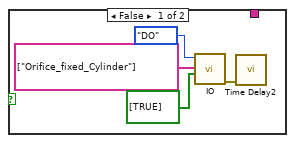
[diagram p8: hidden frame]
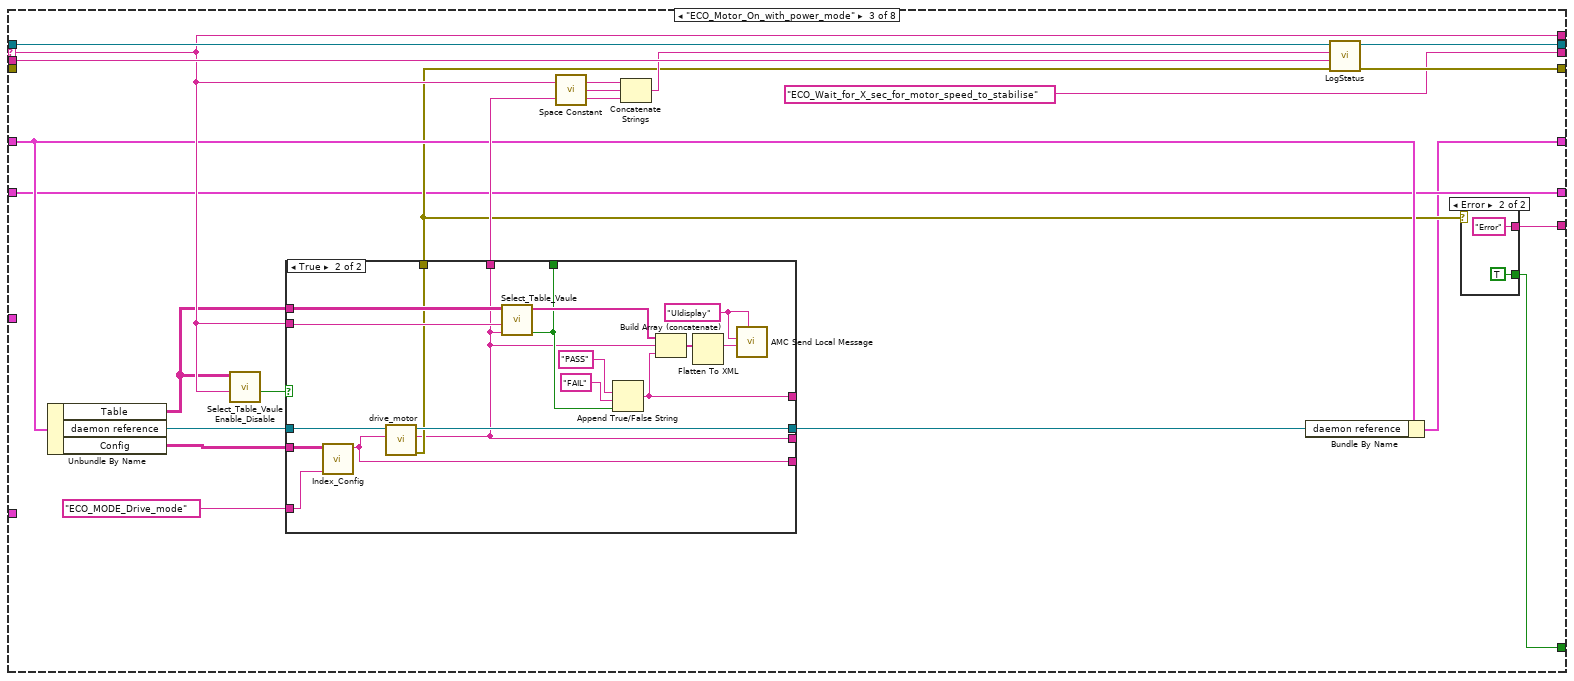
[diagram p9: hidden frame]
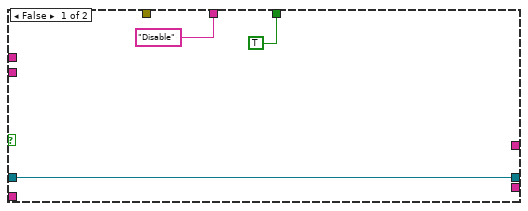
[diagram p11: hidden frame]
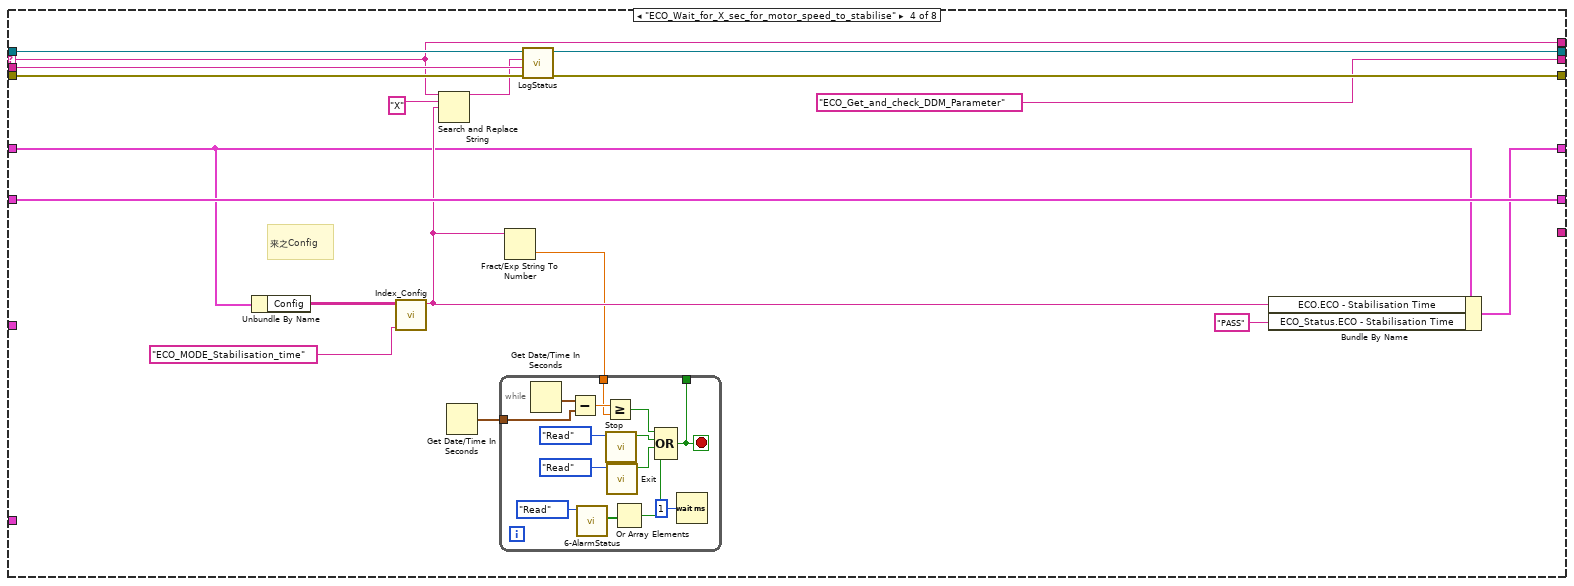
[diagram p12: hidden frame]
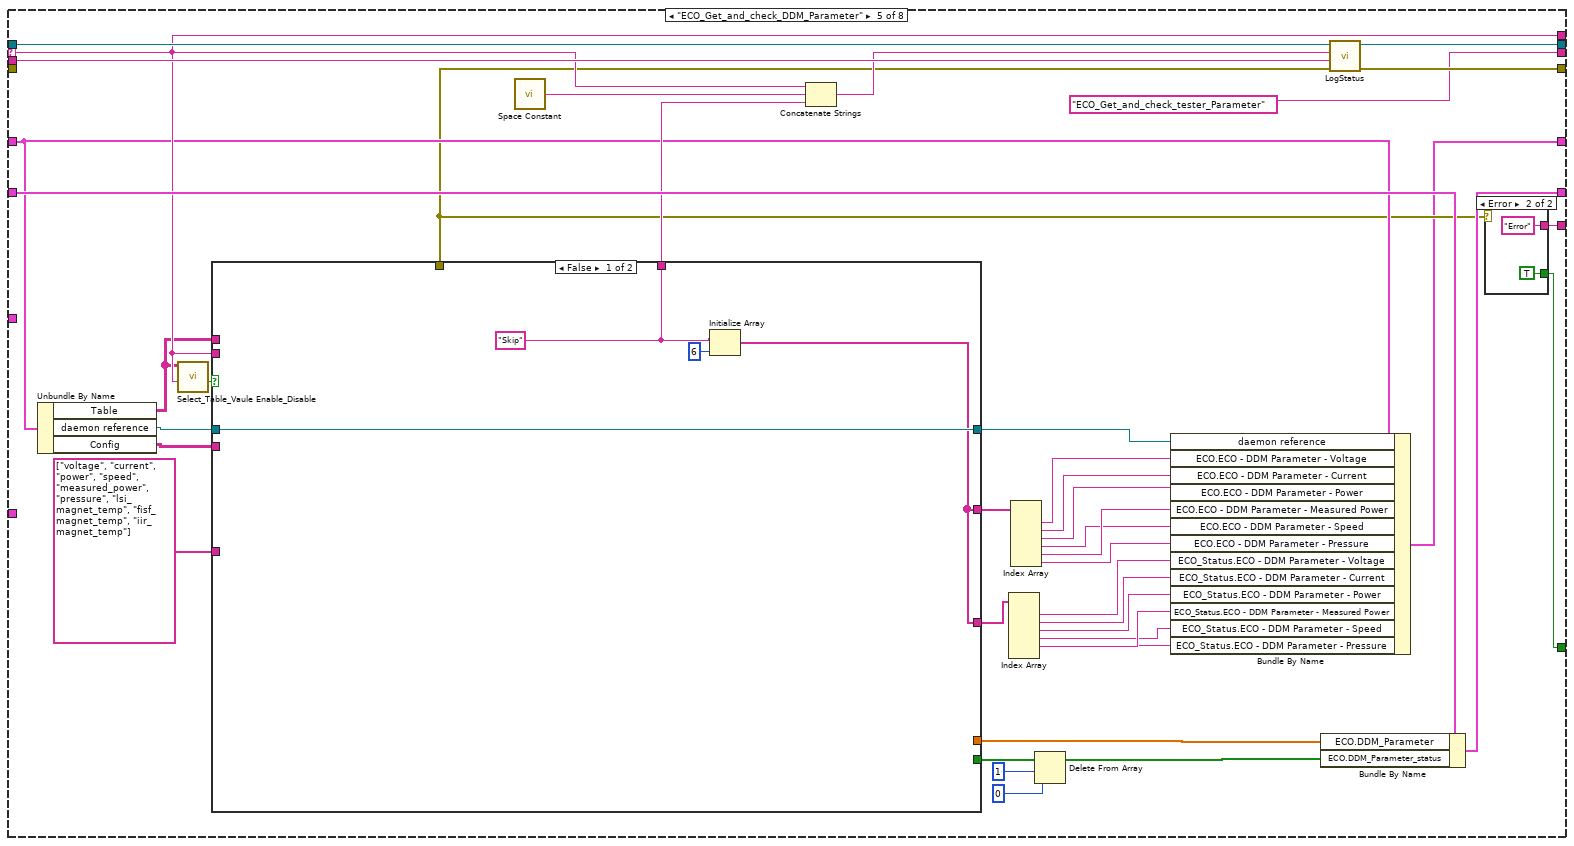
[diagram p13: hidden frame]
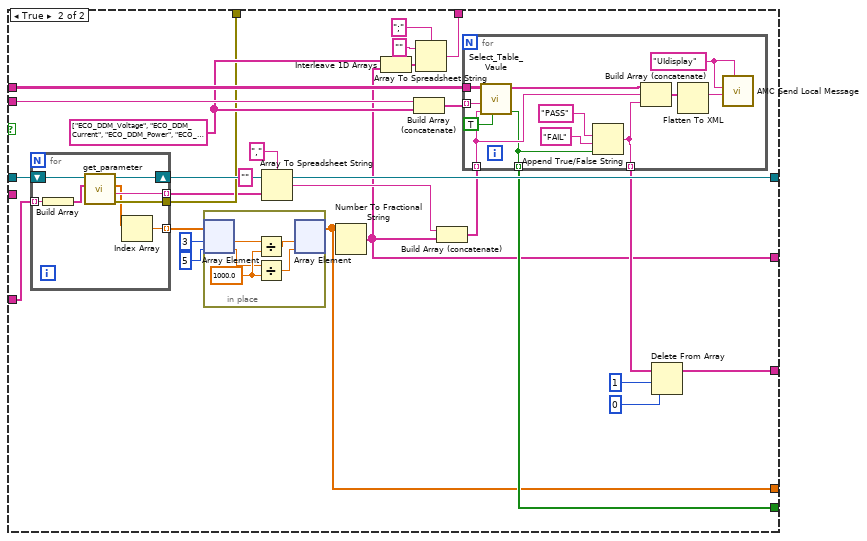
[diagram p15: hidden frame]
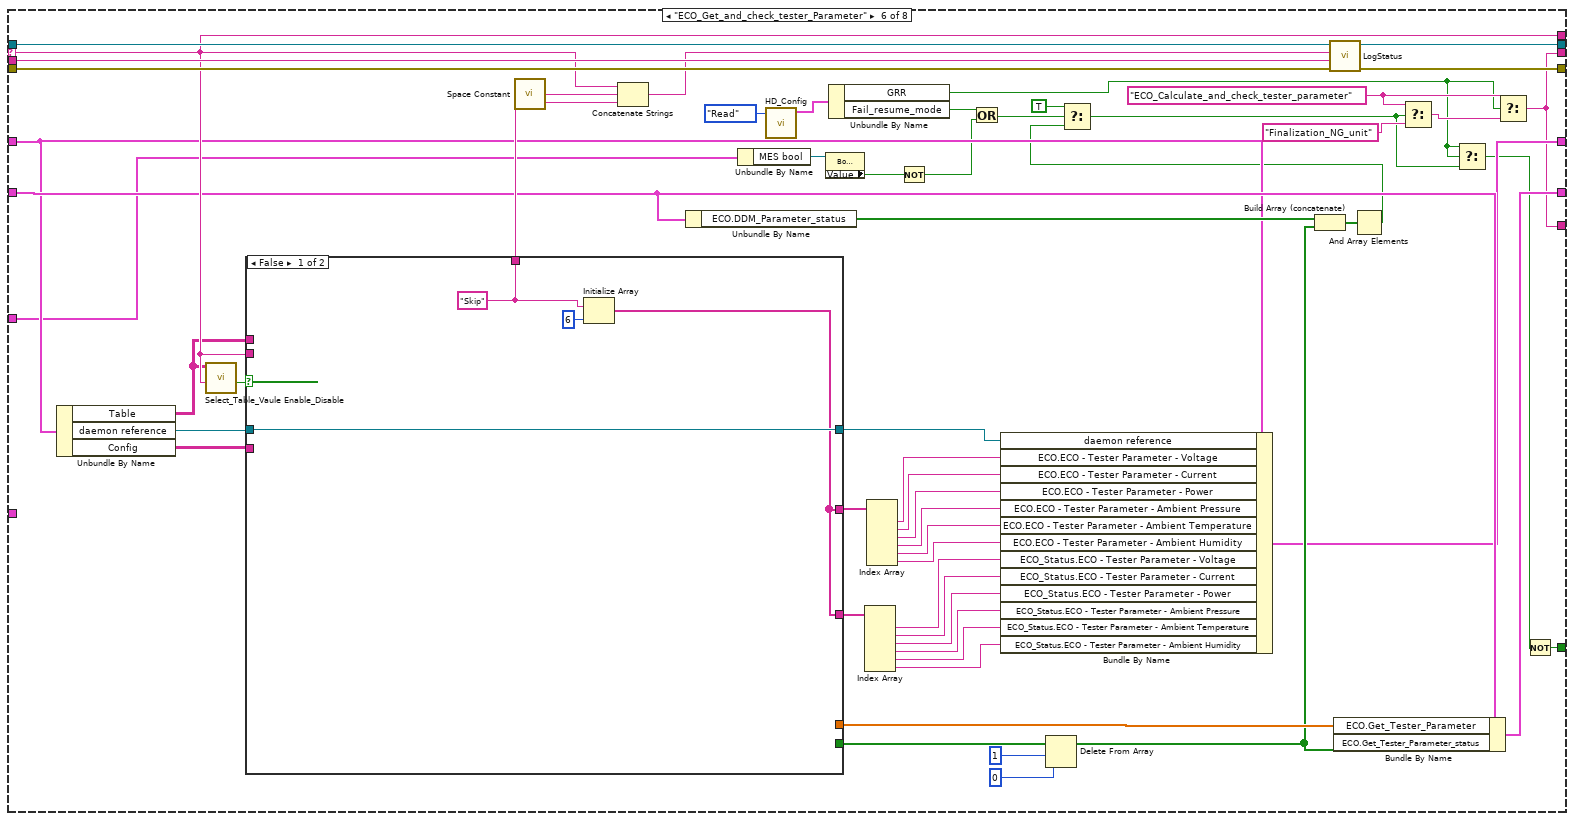
[diagram p16: hidden frame]
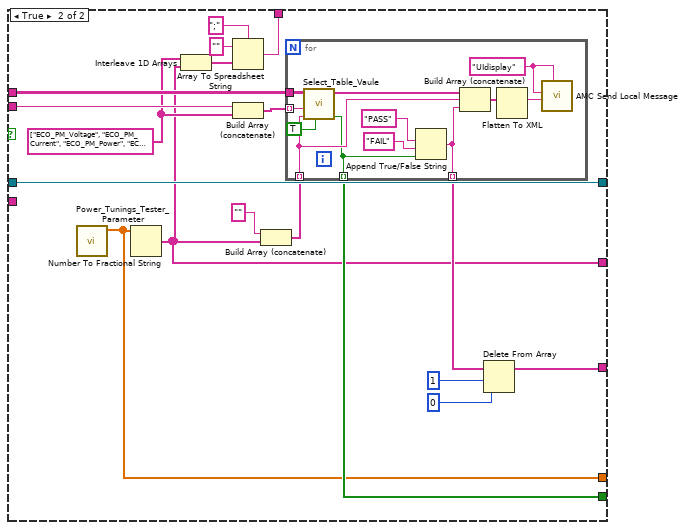
[diagram p17: hidden frame]
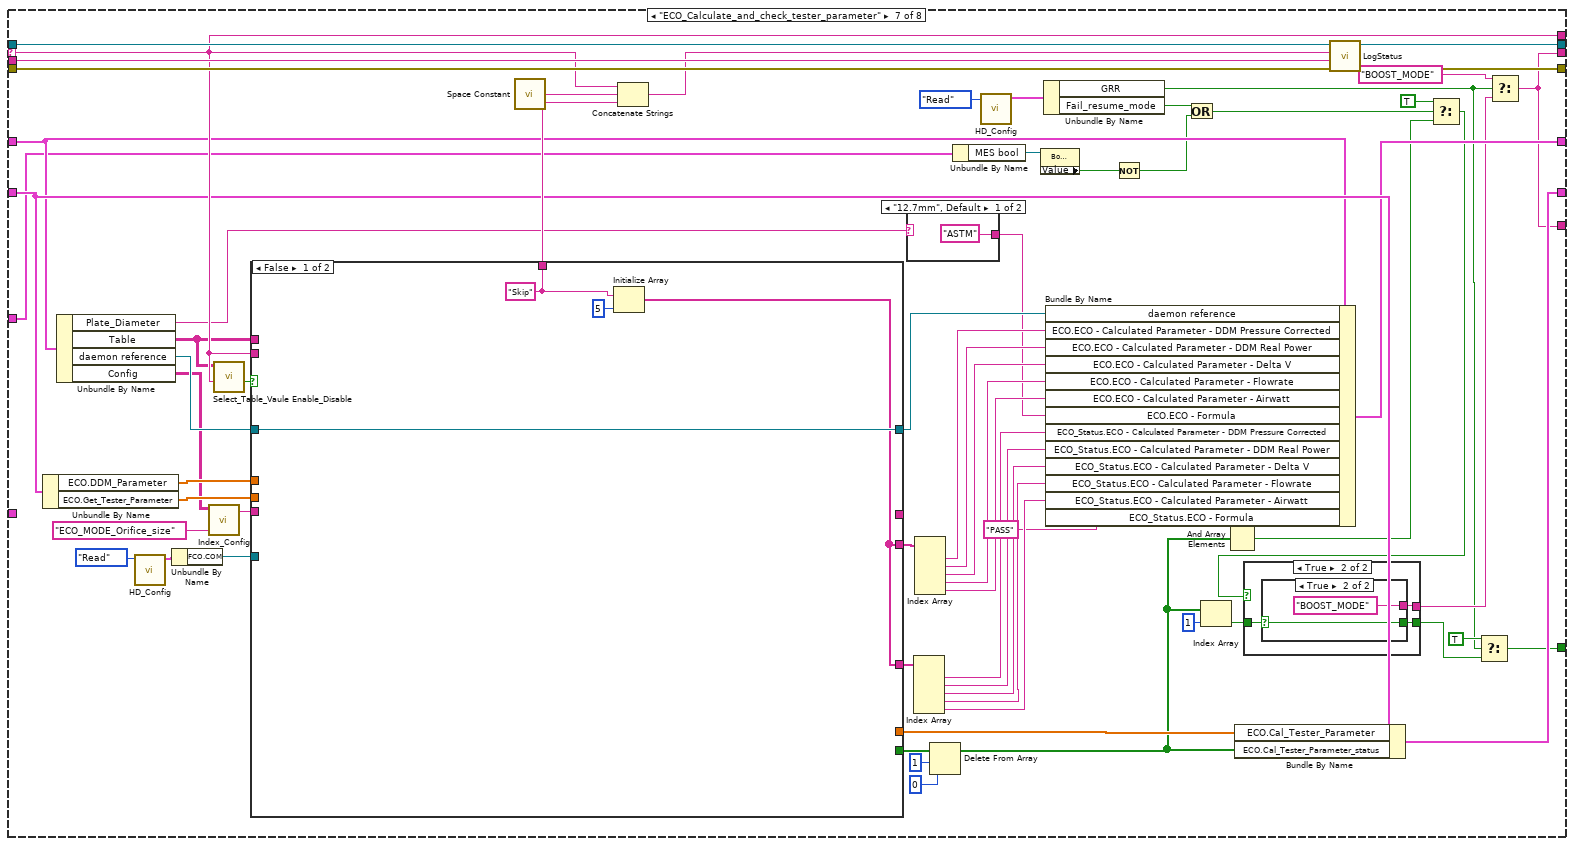
[diagram p18: hidden frame]
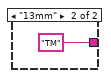
[diagram p19: hidden frame]
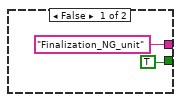
[diagram p20: hidden frame]
diagram:
  n1 = Flush Queue(queue="Message Queue out") -> (queue out=w4:T4)  [unwired: 1 in, 2 out]
  n2 = call "HD_Config.vi"("Step"=enum16{"Initial", "Write", "Read"}."Read") -> ("HD Config out"=w8:T5)  [unwired: 9 in, 1 out]
  n3 = call "AMC Send Local Message.vi"("error in (no error)"="error in (no error)", "Message Name"="ECO_Orifice_Size", "Message Queue in"=w4) -> ("error out"=w13:errorcluster, "Message Queue out"=w14:T4)  [unwired: 7 in]
  n4 = while {
    tunnel: w14 -> [w47]
    tunnel: [w43] -> w6
    tunnel: w13 -> [w41]
    tunnel: [w38] -> w5
    shift-right: [w34] -> w10
    shift-left: "?" -> [w35]
    tunnel: w8 -> [w33]
    tunnel: [w29] -> w7
    shift-right: [w20] -> w2
    shift-left: "Data in" -> [w21]
    tunnel: "AllControls In" -> [w22]
    stop <- w23 stop-if-true
    n5 = Wait (ms)(milliseconds to wait=u32 1 ("等待时间（毫秒）")) -> ()  [unwired: 1 out]
    n6 = call "AMC Read Next Message.vi"("error in (no error)"=w41, "timeout (1ms)"=100, "Message Queue in"=w47) -> ("error out"=w40:errorcluster, "Message Value"=w31:string, "Message Name"=w45:string, "Message Queue out"=w46:T4)  [unwired: 1 in, 4 out]
    n7 = case shown="\"ECO_Power_Tune\"" w45 {
      selector: w45 -> [_ w80 w138 w178 w229 w343 w442 w519]
      tunnel: w46 -> [w51 w84 w145 w184 w238 w352 w450 w534]
      tunnel: [w51 w84 w145 w184 w238 w352 w450 w514] -> w44
      tunnel: w40 -> [w50 w83 _ w183 _ w351 w449 w538]
      tunnel: [w50 w82 w144 w182 w237 w350 w448 w535] -> w39
      tunnel: [_ w58 w132 _ w218 w334 w401 TRUE] -> w24
      tunnel: w35 -> [w49 w55 w128 w176 w234 w337 w440 w530]
      tunnel: [w49 w55 w128 w176 w233 w347 w446 w532] -> w34
      tunnel: w31 -> [_ w81 w143 w181 w236 w349 w447 w537]
      tunnel: [_ w80 w138 w178 w229 w343 w442 w519] -> w30
      tunnel: w33 -> [_ w67 _ _ _ _ _ _]
      tunnel: [_ "ECO_Motor_On_with_power_mode" "ECO_Wait_for_X_sec_for_motor_speed_to_stabilise" "ECO_Get_and_check_DDM_Parameter" "ECO_Get_and_check_tester_Parameter" w313 w408 w531] -> w32
      tunnel: [_ w54 w133 _ w219 w313 w408 w531] -> w29
      tunnel: w22 -> [_ _ _ _ _ w317 w411 w504]
      tunnel: w21 -> [w48 w53 w130 w171 w216 w329 w423 w506]
      tunnel: [w48 w56 w126 w173 w213 w326 w420 w505] -> w20
      frame "假", Default {
      }
      frame "ECO_Orifice_Size" {
        n8 = Unbundle By Name(w67) -> ("Motor.COM"=w73:refnum<visa-resource-name>)
        n9 = Unbundle By Name(w53) -> ("Config"=w72:string[][])
        n10 = call "Position_Config.vi"("Step"=enum16{"Initial", "Write", "Read"}."Read") -> ("Position Config out"=w69:T8)  [unwired: 9 in, 1 out]
        n11 = call "Index_Config.vi"("Action"="ECO_MODE_Orifice_size", "config"=w72) -> ("data"=w57:string)  [unwired: 9 in]
        n12 = case shown="\"12.7\", Default" w57 {
          tunnel: w69 -> [w88 w90 w92 w94]
          tunnel: [w87 w89 w91 w93] -> w68
          frame "12.7", Default {
            n13 = Unbundle By Name(w88) -> ("OrificeSize_12.7"=w87:i32)
          }
          frame "13" {
            n14 = Unbundle By Name(w90) -> ("OrificeSize_13"=w89:i32)
          }
          frame "30" {
            n15 = Unbundle By Name(w92) -> ("OrificeSize_30"=w91:i32)
          }
          frame "16" {
            n16 = Unbundle By Name(w94) -> ("OrificeSize_16"=w93:i32)
          }
        }
        n17 = call "IO.vi"("DO DATA"=bool[] [FALSE] ("Writel_IO"), "IO Name"=string[] ["Orifice_fixed_Cylinder"], "IO?"=enum16{"DI", "DO"}."DO") -> ("error out"=w66:errorcluster)  [unwired: 6 in, 2 out]
        n18 = To Long Integer(number=w68) -> (32bit integer=w75:i32)
        n19 = call "Time Delay"("error in (no error)"=w66) -> ("error out"=w62:errorcluster)  [unwired: 10 in]
        n20 = call "Pulse.vi"("Pulse"=w75) -> ("Pulse"=w76:string)  [unwired: 10 in]
        n21 = call "Motor Visa.vi"("错误输入（无错误）"=w62, "Command"=w76, "VISA资源名称"=w73) -> ("错误输出"=w77:errorcluster, "VISA资源名称输出"=w78:refnum<visa-resource-name>)  [unwired: 6 in, 1 out]
        n22 = call "ABS.vi"() -> ("绝对模式"=w74:string)  [unwired: 11 in]
        n23 = call "LogStatus.vi"("error in (no error)"=w83, "last message"=w81, "message"=w80) -> ("error  out"=w82:errorcluster)  [unwired: 8 in]
        n24 = call "Motor Visa.vi"("错误输入（无错误）"=w77, "Command"=w74, "VISA资源名称"=w78) -> ("VISA资源名称输出"=w61:refnum<visa-resource-name>)  [unwired: 6 in, 2 out]
        n25 = while {
          tunnel: w61 -> [w124]
          tunnel: [w109] -> w59
          tunnel: [w103] -> w60
          stop <- w114 stop-if-true
          n26 = call "Get Status.vi"() -> ("Command"=w125:string)  [unwired: 11 in]
          n27 = call "Get Alarm  Error Status.vi"() -> ("AlarmStatus"=w117:string, "ErrorStatus"=w118:string)  [unwired: 10 in]
          n28 = call "Motor Visa.vi"("Command"=w125, "VISA资源名称"=w124) -> ("读取缓冲区"=w123:string, "VISA资源名称输出"=w116:refnum<visa-resource-name>)  [unwired: 7 in, 1 out]
          n29 = Wait (ms)(milliseconds to wait=u32 50 ("等待时间（毫秒）")) -> ()  [unwired: 1 out]
          n30 = call "Motor Visa.vi"("Command"=w118, "VISA资源名称"=w116) -> ("读取缓冲区"=w120:string, "VISA资源名称输出"=w121:refnum<visa-resource-name>)  [unwired: 7 in, 1 out]
          n31 = call "6-AlarmStatus.vi"("Step"=enum16{"Initial", "Write", "Read"}."Read") -> ("AlarmValue Out"=w107:bool[])  [unwired: 9 in, 1 out]
          n32 = call "Motor Visa.vi"("Command"=w117, "VISA资源名称"=w121) -> ("读取缓冲区"=w119:string)  [unwired: 7 in, 2 out]
          n33 = Or Array Elements(Boolean array=w107) -> (logical OR=w106:bool)
          n34 = call "Exit.vi"("Step"=enum16{"Initial", "Write", "Read"}."Read" ("step")) -> ("Exit Out"=w105:bool)  [unwired: 9 in, 1 out]
          n35 = call "Stop.vi"("Step"=enum16{"Initial", "Write", "Read"}."Read") -> ("Stop Out"=w104:bool)  [unwired: 9 in, 1 out]
          n36 = call "Alarm and Error Result.vi"("Command"=w119) -> ("Alarm or Error"=w111:bool)  [unwired: 10 in]
          n37 = call "Alarm and Error Result.vi"("Command"=w120) -> ("Alarm or Error"=w110:bool)  [unwired: 10 in]
          n38 = call "Motion Down.vi"("Command"=w123) -> ("Motion Down"=w115:bool)  [unwired: 10 in]
          n39 = Or(x=w111, y=w110) -> (x .or. y?=w109:bool)
          n40 = Compound Arithmetic op=OR(w106, w105, w104) -> (w103:bool)
          n41 = Compound Arithmetic op=OR(w106, w105, w104, w111, w110, w115) -> (w114:bool)
        }
        n42 = Or(x=w60, y=w59) -> (x .or. y?=w58:bool)
        n43 = case shown="True" w60 {
          tunnel: w61 -> [_ w86]
          frame False {
          }
          frame True {
            n44 = call "Stop Command.vi"() -> ("Stop"=w85:string)  [unwired: 11 in]
            n45 = call "Motor Visa.vi"("Command"=w85, "VISA资源名称"=w86) -> ()  [unwired: 7 in, 3 out]
          }
        }
        n46 = Bundle By Name(cluster=w53, "ECO.Restriction Plate Diameter"=w57, "ECO_Status.Restriction Plate Diameter"="PASS") -> (w56:T2)
        n47 = case shown="True" w59 {
          tunnel: [_ "Error" ("Message Name")] -> w54
          frame False {
            n48 = call "IO.vi"("DO DATA"=bool[] [TRUE] ("Writel_IO"), "IO Name"=string[] ["Orifice_fixed_Cylinder"], "IO?"=enum16{"DI", "DO"}."DO") -> ("error out"=w95:errorcluster)  [unwired: 6 in, 2 out]
            n49 = call "Time Delay2"("error in (no error)"=w95) -> ()  [unwired: 10 in, 1 out]
          }
          frame True {
            n50 = call "6-AlarmStatus.vi"("AlarmValue"=TRUE, "AlarmIndex"=AlarmIndex."Motor Error", "Step"=enum16{"Initial", "Write", "Read"}."Write") -> ()  [unwired: 7 in, 2 out]
          }
        }
      }
      frame "ECO_Motor_On_with_power_mode" {
        n51 = Unbundle By Name(w130) -> ("Table"=w137:string[][], "daemon reference"=w142:refnum<k5>, "Config"=w135:string[][])
        n52 = call "Select_Table_Vaule Enable_Disable.vi"("Action"=w138, "Table"=w137) -> ("Enable"=w139:bool)  [unwired: 8 in, 1 out]
        n53 = case shown="True" w139 {
          tunnel: w142 -> [w149 w167]
          tunnel: [TRUE w157] -> _
          tunnel: [w149 w161] -> w127
          tunnel: ["Disable" ("response") w153] -> w131
          tunnel: w138 -> [_ w160]
          tunnel: w137 -> [_ w159]
          tunnel: w135 -> [_ w156]
          tunnel: "ECO_MODE_Drive_mode" -> [_ w155]
          tunnel: [_ w154] -> w129
          tunnel: [_ w153] -> _
          tunnel: [_ w152] -> _
          tunnel: [_ w151] -> _
          frame False {
          }
          frame True {
            w166 = "UIdisplay" ("Process (\"\" - local)")
            n54 = call "Index_Config.vi"("Action"=w155, "config"=w156) -> ("data"=w151:string)  [unwired: 9 in]
            n55 = call "drive_motor.vi"("Power Mode"=w151, "daemon reference in"=w167) -> ("error out"=w154:errorcluster, "response"=w153:string, "daemon reference out"=w161:refnum<k5>)  [unwired: 6 in, 1 out]
            n56 = call "Select_Table_Vaule.vi"("Vaule"=w153, "Action"=w160, "Table"=w159) -> ("Result"=w157:bool, "vaule"=w158:string[])  [unwired: 7 in]
            n57 = Append True/False String(1:w157, 2:"FAIL" ("真字符串"), 3:"PASS" ("真字符串")) -> (0:w152:string)  [unwired: 1 in]
            n58 = Build Array (concatenate)(w158, w153, w152) -> (w165:string[])
            n59 = Flatten To XML(anything=w165) -> (xml string=w164:string)
            n60 = call "AMC Send Local Message.vi"("Process (\"\" - local)"=w166, "Message Value"=w164, "Message Name"=w166) -> ()  [unwired: 7 in, 2 out]
          }
        }
        n61 = call <vilib>:"Space Constant.vi"() -> ("String"=w141:string)
        n62 = Concatenate Strings(w138, w141, w131) -> (w140:string)
        n63 = Bundle By Name(cluster=w130, "daemon reference"=w127) -> (w126:T2)
        n64 = call "LogStatus.vi"("error in (no error)"=w129, "last message"=w143, "message"=w140) -> ("error  out"=w144:errorcluster)  [unwired: 8 in]
        n65 = case shown="Error" w129 {
          tunnel: [_ TRUE] -> w132
          tunnel: [_ "Error"] -> w133
          frame No Error {
          }
          frame Error {
          }
        }
      }
      frame "ECO_Wait_for_X_sec_for_motor_speed_to_stabilise" {
        # "来之Config"
        n66 = Unbundle By Name(w171) -> ("Config"=w175:string[][])
        n67 = call "Index_Config.vi"("Action"="ECO_MODE_Stabilisation_time", "config"=w175) -> ("data"=w172:string)  [unwired: 9 in]
        n68 = Search and Replace String(input string=w178, search string="X" ("搜索字符串"), replace string=w172) -> (result string=w179:string)  [unwired: 5 in, 3 out]
        n69 = Get Date/Time In Seconds() -> (seconds since 1Jan1904=w170:timestamp)
        n70 = Fract/Exp String To Number(string=w172) -> (number=w169:dbl)  [unwired: 3 in, 1 out]
        n71 = while {
          tunnel: w170 -> [w191]
          tunnel: w169 -> [w188]
          tunnel: [w187] -> _
          stop <- w187 stop-if-true
          n72 = Get Date/Time In Seconds() -> (seconds since 1Jan1904=w192:timestamp)
          n73 = Subtract(x=w192, y=w191) -> (x-y=w190:dbl)
          n74 = call "6-AlarmStatus.vi"("Step"=enum16{"Initial", "Write", "Read"}."Read") -> ("AlarmValue Out"=w195:bool[])  [unwired: 9 in, 1 out]
          n75 = Greater Or Equal?(x=w190, y=w188) -> (x >= y?=w189:bool)
          n76 = call "Stop.vi"("Step"=enum16{"Initial", "Write", "Read"}."Read") -> ("Stop Out"=w193:bool)  [unwired: 9 in, 1 out]
          n77 = call "Exit.vi"("Step"=enum16{"Initial", "Write", "Read"}."Read" ("step")) -> ("Exit Out"=w197:bool)  [unwired: 9 in, 1 out]
          n78 = Or Array Elements(Boolean array=w195) -> (logical OR=w194:bool)
          n79 = Compound Arithmetic op=OR(w189, w193, w197, w194) -> (w187:bool)
          n80 = Wait (ms)(milliseconds to wait=u32 1 ("等待时间（毫秒）")) -> ()  [unwired: 1 out]
        }
        n81 = call "LogStatus.vi"("error in (no error)"=w183, "last message"=w181, "message"=w179) -> ("error  out"=w182:errorcluster)  [unwired: 8 in]
        n82 = Bundle By Name(cluster=w171, "ECO.ECO - Stabilisation Time"=w172, "ECO_Status.ECO - Stabilisation Time"="PASS") -> (w173:T2)
      }
      frame "ECO_Get_and_check_DDM_Parameter" {
        n83 = Unbundle By Name(w216) -> ("Table"=w228:string[][], "daemon reference"=w235:refnum<k5>, "Config"=w226:string[][])
        n84 = call "Select_Table_Vaule Enable_Disable.vi"("Action"=w229, "Table"=w228) -> ("Enable"=w227:bool)  [unwired: 8 in, 1 out]
        n85 = case shown="False" w227 {
          tunnel: w235 -> [w244 w270]
          tunnel: [w244 w269] -> w214
          tunnel: [w243 w263] -> w230
          tunnel: w229 -> [_ w266]
          tunnel: w228 -> [_ w271]
          tunnel: w226 -> [_ _]
          tunnel: [_ w255] -> w224
          tunnel: [_ w268] -> w223
          tunnel: [_ w259] -> w215
          tunnel: T7[] ["voltage", "current", "power", "speed", "measured_power", "pressure", "lsi_magnet_temp", "fisf_magnet_temp", "iir_magnet_temp"] ("Parameter") -> [_ w254]
          tunnel: [w242 w246] -> w212
          tunnel: [w242 w245] -> w205
          frame False {
            w243 = "Skip" ("software string")
            n86 = Initialize Array(w243, 6 ("维数大小")) -> (w242:string[])
          }
          frame True {
            w264 = string[] ["ECO_DDM_Voltage", "ECO_DDM_Current", "ECO_DDM_Power", "ECO_DDM_Speed", "ECO_DDM_Measured_Power", "ECO_DDM_Pressure", "ECO_lsi_magnet_temp", "ECO_fisf_magnet_temp", "ECO_iir_magnet_temp"]
            n87 = for {
              tunnel: [w277] -> w253 mode=indexing
              tunnel: [w276] -> w259
              tunnel: [w272] -> w256 mode=indexing
              tunnel: w254 -> [w274] mode=indexing
              shift-right: [w278] -> w269
              shift-left: w270 -> [w279]
              n88 = Build Array(w274) -> (w273:T7[])
              n89 = call "get_parameter.vi"("Parameter"=w273, "daemon reference in"=w279) -> ("error out"=w276:errorcluster, "response"=w277:string, "values"=w275:dbl[], "daemon reference out"=w278:refnum<k5>)  [unwired: 5 in, 1 out]
              n90 = Index Array(array=w275) -> (element=w272:dbl)  [unwired: 1 in]
            }
            n91 = in-place {
              w284 = 1000.0
              n92 = in-place-array #1(w256, 3, 5) -> (w283:dbl, w280:dbl)
              n93 = Divide(x=w283, y=w284) -> (x/y=w282:dbl)
              n94 = Divide(x=w280, y=w284) -> (x/y=w281:dbl)
              n95 = in-place-array #1(w282, w281) -> (w255:dbl[])  [unwired: 2 out]
            }
            n96 = Array To Spreadsheet String(delimiter (Tab)=",", array=w253, 3:"" ("format string")) -> (spreadsheet string=w252:string)
            n97 = Number To Fractional String(number=w255) -> (F-format string=w246:string[])  [unwired: 3 in]
            n98 = Interleave 1D Arrays(w264, w246) -> (w260:string[])
            n99 = Build Array (concatenate)(w266, w264) -> (w267:string[])
            n100 = Array To Spreadsheet String(delimiter (Tab)=";" ("格式字符串"), array=w260, 3:"" ("格式字符串")) -> (spreadsheet string=w263:string)
            n101 = Build Array (concatenate)(w252, w246) -> (w265:string[])
            n102 = for {
              tunnel: w271 -> [w291]
              tunnel: w265 -> [w289] mode=indexing
              tunnel: w267 -> [w288] mode=indexing
              tunnel: [w287] -> w268 mode=indexing
              tunnel: [w285] -> w247 mode=indexing
              w296 = "UIdisplay" ("Process (\"\" - local)")
              n103 = call "Select_Table_Vaule.vi"("Boolean"=TRUE, "Vaule"=w289, "Action"=w288, "Table"=w291) -> ("Result"=w287:bool, "vaule"=w290:string[])  [unwired: 6 in]
              n104 = Append True/False String(1:w287, 2:"FAIL" ("真字符串"), 3:"PASS" ("真字符串")) -> (0:w285:string)  [unwired: 1 in]
              n105 = Build Array (concatenate)(w290, w289, w285) -> (w295:string[])
              n106 = Flatten To XML(anything=w295) -> (xml string=w294:string)
              n107 = call "AMC Send Local Message.vi"("Process (\"\" - local)"=w296, "Message Value"=w294, "Message Name"=w296) -> ()  [unwired: 7 in, 2 out]
            }
            n108 = Delete From Array(array=w247, length=1 ("长度"), index=0 ("索引")) -> (array with subset deleted=w245:string[])  [unwired: 1 out]
          }
        }
        n109 = call <vilib>:"Space Constant.vi"() -> ("String"=w232:string)
        n110 = Concatenate Strings(w229, w232, w230) -> (w231:string)
        n111 = Index Array(array=w205) -> (element #1=w204:string, element #2=w203:string, element #3=w202:string, element #4=w200:string, element #5=w201:string, element #6=w199:string)  [unwired: 6 in]
        n112 = Index Array(array=w212) -> (element #1=w211:string, element #2=w210:string, element #3=w209:string, element #4=w206:string, element #5=w207:string, element #6=w208:string)  [unwired: 6 in]
        n113 = Delete From Array(array=w223, length=1 ("长度"), index=0 ("索引")) -> (array with subset deleted=w222:bool[])  [unwired: 1 out]
        n114 = Bundle By Name(cluster=w216, "daemon reference"=w214, "ECO.ECO - DDM Parameter - Voltage"=w211, "ECO.ECO - DDM Parameter - Current"=w210, "ECO.ECO - DDM Parameter - Power"=w209, "ECO.ECO - DDM Parameter - Measured Power"=w207, "ECO.ECO - DDM Parameter - Speed"=w206, "ECO.ECO - DDM Parameter - Pressure"=w208, "ECO_Status.ECO - DDM Parameter - Voltage"=w204, "ECO_Status.ECO - DDM Parameter - Current"=w203, "ECO_Status.ECO - DDM Parameter - Power"=w202, "ECO_Status.ECO - DDM Parameter - Measured Power"=w201, "ECO_Status.ECO - DDM Parameter - Speed"=w200, "ECO_Status.ECO - DDM Parameter - Pressure"=w199) -> (w213:T2)
        n115 = Bundle By Name(cluster=w234, "ECO.DDM_Parameter"=w224, "ECO.DDM_Parameter_status"=w222) -> (w233:T3)
        n116 = call "LogStatus.vi"("error in (no error)"=w215, "last message"=w236, "message"=w231) -> ("error  out"=w237:errorcluster)  [unwired: 8 in]
        n117 = case shown="Error" w215 {
          tunnel: [_ TRUE] -> w218
          tunnel: [_ "Error"] -> w219
          frame No Error {
          }
          frame Error {
          }
        }
      }
      frame "ECO_Get_and_check_tester_Parameter" {
        w314 = "ECO_Calculate_and_check_tester_parameter"
        n118 = Unbundle By Name(w329) -> ("Table"=w342:string[][], "daemon reference"=w348:refnum<k5>, "Config"=w340:string[][])
        n119 = call "Select_Table_Vaule Enable_Disable.vi"("Action"=w343, "Table"=w342) -> ("Enable"=w341:bool)  [unwired: 8 in, 1 out]
        n120 = case shown="False" w341 {
          tunnel: w348 -> [w356 w373]
          tunnel: [w356 w373] -> w327
          tunnel: [w355 w363] -> w344
          tunnel: w343 -> [_ w370]
          tunnel: w342 -> [_ w374]
          tunnel: w340 -> [_ _]
          tunnel: [_ w362] -> w339
          tunnel: [_ w372] -> w333
          tunnel: [w354 w358] -> w303
          tunnel: [w354 w357] -> w328
          frame False {
            w355 = "Skip" ("software string")
            n121 = Initialize Array(w355, 6 ("维数大小")) -> (w354:string[])
          }
          frame True {
            w364 = string[] ["ECO_PM_Voltage", "ECO_PM_Current", "ECO_PM_Power", "ECO_Ambient_Pressure", "ECO_Ambient_Temperature", "ECO_Ambient_humidity", "ECO_Tester_Reference_Ambient_Pressure"]
            n122 = call "Power_Tunings_Tester_Parameter.vi"() -> ("Power_Tuning_Tester_Parameter"=w362:dbl[])  [unwired: 11 in]
            n123 = Number To Fractional String(number=w362) -> (F-format string=w357:string[])  [unwired: 3 in]
            n124 = Interleave 1D Arrays(w364, w357) -> (w365:string[])
            n125 = Array To Spreadsheet String(delimiter (Tab)=";" ("格式字符串"), array=w365, 3:"" ("格式字符串")) -> (spreadsheet string=w363:string)
            n126 = Build Array (concatenate)(w370, w364) -> (w371:string[])
            n127 = Build Array (concatenate)("", w357) -> (w369:string[])
            n128 = for {
              tunnel: w374 -> [w381]
              tunnel: w369 -> [w379] mode=indexing
              tunnel: w371 -> [w378] mode=indexing
              tunnel: [w377] -> w372 mode=indexing
              tunnel: [w375] -> w359 mode=indexing
              w386 = "UIdisplay" ("Process (\"\" - local)")
              n129 = call "Select_Table_Vaule.vi"("Boolean"=TRUE, "Vaule"=w379, "Action"=w378, "Table"=w381) -> ("Result"=w377:bool, "vaule"=w380:string[])  [unwired: 6 in]
              n130 = Append True/False String(1:w377, 2:"FAIL" ("真字符串"), 3:"PASS" ("真字符串")) -> (0:w375:string)  [unwired: 1 in]
              n131 = Build Array (concatenate)(w380, w379, w375) -> (w385:string[])
              n132 = Flatten To XML(anything=w385) -> (xml string=w384:string)
              n133 = call "AMC Send Local Message.vi"("Process (\"\" - local)"=w386, "Message Value"=w384, "Message Name"=w386) -> ()  [unwired: 7 in, 2 out]
            }
            n134 = Delete From Array(array=w359, length=1 ("长度"), index=0 ("索引")) -> (array with subset deleted=w358:string[])  [unwired: 1 out]
          }
        }
        n135 = call <vilib>:"Space Constant.vi"() -> ("String"=w346:string)
        n136 = Concatenate Strings(w343, w346, w344) -> (w345:string)
        n137 = Unbundle By Name(w337) -> ("ECO.DDM_Parameter_status"=w336:bool[])
        n138 = Unbundle By Name(w317) -> ("MES bool"=w321:refnum<vi>)
        n139 = call "HD_Config.vi"("Step"=enum16{"Initial", "Write", "Read"}."Read") -> ("HD Config out"=w320:T5)  [unwired: 9 in, 1 out]
        n140 = property class="Bool (严格)"(reference=w321) -> ("Value"=w323:bool)  [unwired: 1 in, 2 out]
        n141 = Unbundle By Name(w320) -> ("GRR"=w312:bool, "Fail_resume_mode"=w322:bool)
        n142 = Index Array(array=w303) -> (element #1=w302:string, element #2=w301:string, element #3=w300:string, element #4=w299:string, element #5=w298:string, element #6=w297:string)  [unwired: 6 in]
        n143 = Index Array(array=w328) -> (element #1=w309:string, element #2=w308:string, element #3=w307:string, element #4=w306:string, element #5=w305:string, element #6=w304:string)  [unwired: 6 in]
        n144 = Not(x=w323) -> (.not. x?=w325:bool)
        n145 = Or(x=w322, y=w325) -> (x .or. y?=w324:bool)
        n146 = Bundle By Name(cluster=w329, "daemon reference"=w327, "ECO.ECO - Tester Parameter - Voltage"=w309, "ECO.ECO - Tester Parameter - Current"=w308, "ECO.ECO - Tester Parameter - Power"=w307, "ECO.ECO - Tester Parameter - Ambient Pressure"=w306, "ECO.ECO - Tester Parameter - Ambient Temperature"=w305, "ECO.ECO - Tester Parameter - Ambient Humidity"=w304, "ECO_Status.ECO - Tester Parameter - Voltage"=w302, "ECO_Status.ECO - Tester Parameter - Current"=w301, "ECO_Status.ECO - Tester Parameter - Power"=w300, "ECO_Status.ECO - Tester Parameter - Ambient Pressure"=w299, "ECO_Status.ECO - Tester Parameter - Ambient Temperature"=w298, "ECO_Status.ECO - Tester Parameter - Ambient Humidity"=w297) -> (w326:T2)
        n147 = Delete From Array(array=w333, length=1 ("长度"), index=0 ("索引")) -> (array with subset deleted=w332:bool[])  [unwired: 1 out]
        n148 = Build Array (concatenate)(w336, w332) -> (w335:bool[])
        n149 = call "LogStatus.vi"("error in (no error)"=w351, "last message"=w349, "message"=w345) -> ("error  out"=w350:errorcluster)  [unwired: 8 in]
        n150 = Bundle By Name(cluster=w337, "ECO.Get_Tester_Parameter"=w339, "ECO.Get_Tester_Parameter_status"=w332) -> (w347:T3)
        n151 = And Array Elements(Boolean array=w335) -> (logical AND=w316:bool)
        n152 = Select(t=TRUE, s=w324, f=w316) -> (s? t:f=w311:bool)
        n153 = Select(t=w314, s=w311, f="Finalization_NG_unit") -> (s? t:f=w315:string)
        n154 = Select(t=w312, s=w312, f=w311) -> (s? t:f=w310:bool)
        n155 = Select(t=w314, s=w312, f=w315) -> (s? t:f=w313:string)
        n156 = Not(x=w310) -> (.not. x?=w334:bool)
      }
      frame "ECO_Calculate_and_check_tester_parameter" {
        n157 = Unbundle By Name(w440) -> ("ECO.DDM_Parameter"=w432:dbl[], "ECO.Get_Tester_Parameter"=w431:dbl[])
        n158 = Unbundle By Name(w423) -> ("Plate_Diameter"=w387:string, "Table"=w426:string[][], "daemon reference"=w425:refnum<k5>, "Config"=w424:string[][])
        n159 = call "HD_Config.vi"("Step"=enum16{"Initial", "Write", "Read"}."Read") -> ("HD Config out"=w428:T5)  [unwired: 9 in, 1 out]
        n160 = Unbundle By Name(w428) -> ("FCO.COM"=w427:refnum<visa-resource-name>)
        n161 = call "Index_Config.vi"("Action"="ECO_MODE_Orifice_size", "config"=w424) -> ("data"=w430:string)  [unwired: 9 in]
        n162 = call "Select_Table_Vaule Enable_Disable.vi"("Action"=w442, "Table"=w426) -> ("Enable"=w441:bool)  [unwired: 8 in, 1 out]
        n163 = case shown="False" w441 {
          tunnel: w425 -> [w465 w490]
          tunnel: [w465 w490] -> w421
          tunnel: [w464 w480] -> w443
          tunnel: w442 -> [_ w487]
          tunnel: w426 -> [_ w491]
          tunnel: [_ w473] -> w438
          tunnel: [_ w489] -> w437
          tunnel: w432 -> [_ w478]
          tunnel: w431 -> [_ w477]
          tunnel: w430 -> [_ w476]
          tunnel: w427 -> [_ w474]
          tunnel: [w463 w469] -> w394
          tunnel: [_ w467] -> _
          tunnel: [w463 w466] -> w422
          frame False {
            w464 = "Skip" ("software string")
            n164 = Initialize Array(w464, 5 ("维数大小")) -> (w463:string[])
          }
          frame True {
            w481 = string[] ["ECO_DDM_Pressure_corrected", "ECO_DDM_Real_Power", "ECO_Delta_V", "ECO_Flow_rate", "ECO_AW"]
            n165 = call "FCO_Read.vi"("VISA in"=w474) -> ("Pressure(Pa)"=w468:dbl)  [unwired: 7 in, 3 out]
            n166 = Fract/Exp String To Number(string=w476) -> (number=w475:dbl)  [unwired: 3 in, 1 out]
            n167 = Number To Fractional String(number=w468) -> (F-format string=w467:string)  [unwired: 3 in]
            n168 = call "AW_Calculate_Tester_Parameter.vi"("Tester Parameter"=w477, "DDM Parameter"=w478, "AW_Box_Pressure/Stag Total-Static Pressure rise"=w468, "Orifice_Plate_Diameter"=w475) -> ("Calculate Tester Parameter"=w479:dbl[])  [unwired: 7 in]
            n169 = Number To Fractional String(number=w479) -> (F-format string=w466:string[])  [unwired: 3 in]
            n170 = Interleave 1D Arrays(w481, w466) -> (w484:string[])
            n171 = Array To Spreadsheet String(delimiter (Tab)=";" ("格式字符串"), array=w484, 3:"" ("格式字符串")) -> (spreadsheet string=w480:string)
            n172 = Build Array (concatenate)(w487, w481) -> (w488:string[])
            n173 = Build Array (concatenate)("", w466) -> (w486:string[])
            n174 = for {
              tunnel: w491 -> [w498]
              tunnel: w486 -> [w496] mode=indexing
              tunnel: w488 -> [w495] mode=indexing
              tunnel: [w494] -> w489 mode=indexing
              tunnel: [w492] -> w470 mode=indexing
              w503 = "UIdisplay" ("Process (\"\" - local)")
              n175 = call "Select_Table_Vaule.vi"("Boolean"=TRUE, "Vaule"=w496, "Action"=w495, "Table"=w498) -> ("Result"=w494:bool, "vaule"=w497:string[])  [unwired: 6 in]
              n176 = Append True/False String(1:w494, 2:"FAIL" ("真字符串"), 3:"PASS" ("真字符串")) -> (0:w492:string)  [unwired: 1 in]
              n177 = Build Array (concatenate)(w497, w496, w492) -> (w502:string[])
              n178 = Flatten To XML(anything=w502) -> (xml string=w501:string)
              n179 = call "AMC Send Local Message.vi"("Process (\"\" - local)"=w503, "Message Value"=w501, "Message Name"=w503) -> ()  [unwired: 7 in, 2 out]
            }
            n180 = Build Array (concatenate)(w479, w468) -> (w473:dbl[])
            n181 = Delete From Array(array=w470, length=1 ("长度"), index=0 ("索引")) -> (array with subset deleted=w469:string[])  [unwired: 1 out]
          }
        }
        n182 = call <vilib>:"Space Constant.vi"() -> ("String"=w445:string)
        n183 = Concatenate Strings(w442, w445, w443) -> (w444:string)
        n184 = case shown="\"12.7mm\", Default" w387 {
          tunnel: ["ASTM" ("ECO.ECO - Formula") "TM" ("ECO.ECO - Formula")] -> w395
          frame "12.7mm", Default {
          }
          frame "13mm" {
          }
        }
        n185 = Index Array(array=w394) -> (element #1=w393:string, element #2=w392:string, element #3=w391:string, element #4=w390:string, element #5=w389:string)  [unwired: 5 in]
        n186 = Index Array(array=w422) -> (element #1=w400:string, element #2=w399:string, element #3=w398:string, element #4=w397:string, element #5=w396:string)  [unwired: 5 in]
        n187 = Delete From Array(array=w437, length=1 ("长度"), index=0 ("索引")) -> (array with subset deleted=w436:bool[])  [unwired: 1 out]
        n188 = Unbundle By Name(w411) -> ("MES bool"=w415:refnum<vi>)
        n189 = call "HD_Config.vi"("Step"=enum16{"Initial", "Write", "Read"}."Read") -> ("HD Config out"=w414:T5)  [unwired: 9 in, 1 out]
        n190 = property class="Bool (严格)"(reference=w415) -> ("Value"=w417:bool)  [unwired: 1 in, 2 out]
        n191 = Unbundle By Name(w414) -> ("GRR"=w402:bool, "Fail_resume_mode"=w416:bool)
        n192 = Bundle By Name(cluster=w423, "daemon reference"=w421, "ECO.ECO - Calculated Parameter - DDM Pressure Corrected"=w400, "ECO.ECO - Calculated Parameter - DDM Real Power"=w399, "ECO.ECO - Calculated Parameter - Delta V"=w398, "ECO.ECO - Calculated Parameter - Flowrate"=w397, "ECO.ECO - Calculated Parameter - Airwatt"=w396, "ECO.ECO - Formula"=w395, "ECO_Status.ECO - Calculated Parameter - DDM Pressure Corrected"=w393, "ECO_Status.ECO - Calculated Parameter - DDM Real Power"=w392, "ECO_Status.ECO - Calculated Parameter - Delta V"=w391, "ECO_Status.ECO - Calculated Parameter - Flowrate"=w390, "ECO_Status.ECO - Calculated Parameter - Airwatt"=w389, "ECO_Status.ECO - Formula"="PASS") -> (w420:T2)
        n193 = Not(x=w417) -> (.not. x?=w419:bool)
        n194 = Or(x=w416, y=w419) -> (x .or. y?=w418:bool)
        n195 = Index Array(array=w436, index=1 ("索引")) -> (element=w405:bool)
        n196 = And Array Elements(Boolean array=w436) -> (logical AND=w410:bool)
        n197 = Bundle By Name(cluster=w440, "ECO.Cal_Tester_Parameter"=w438, "ECO.Cal_Tester_Parameter_status"=w436) -> (w446:T3)
        n198 = call "LogStatus.vi"("error in (no error)"=w449, "last message"=w447, "message"=w444) -> ("error  out"=w448:errorcluster)  [unwired: 8 in]
        n199 = Select(t=TRUE, s=w418, f=w410) -> (s? t:f=w407:bool)
        n200 = case shown="True" w407 {
          tunnel: ["Finalization_NG_unit" w457] -> w406
          tunnel: w405 -> [_ w456]
          tunnel: [TRUE w455] -> w403
          frame False {
          }
          frame True {
            n201 = case shown="True" w456 {
              selector: w456 -> [w458 w460]
              tunnel: ["ECO_Power_Tune" "BOOST_MODE"] -> w457
              tunnel: [w458 w460] -> w455
              frame False {
              }
              frame True {
              }
            }
          }
        }
        n202 = Select(t=TRUE, s=w402, f=w403) -> (s? t:f=w401:bool)
        n203 = Select(t="BOOST_MODE", s=w402, f=w406) -> (s? t:f=w408:string)
      }
      frame "ECO_Power_Tune" {
        w521 = "UIdisplay" ("Process (\"\" - local)")
        n204 = Unbundle By Name(w504) -> ("MES bool"=w510:refnum<vi>)
        n205 = call "HD_Config.vi"("Step"=enum16{"Initial", "Write", "Read"}."Read") -> ("HD Config out"=w509:T5)  [unwired: 9 in, 1 out]
        n206 = Unbundle By Name(w506) -> ("Table"=w520:string[][])
        n207 = property class="Bool (严格)"(reference=w510) -> ("Value"=w512:bool)  [unwired: 1 in, 2 out]
        n208 = Unbundle By Name(w509) -> ("Fail_resume_mode"=w511:bool)
        n209 = Not(x=w512) -> (.not. x?=w513:bool)
        n210 = call "Select_Table_Vaule Enable_Disable.vi"("Action"=w519, "Table"=w520) -> ("Enable"=w516:bool)  [unwired: 8 in, 1 out]
        n211 = Or(x=w511, y=w513) -> (x .or. y?=w507:bool)
        n212 = call "LogStatus.vi"("error in (no error)"=w538, "last message"=w537, "message"=w519) -> ("error  out"=w536:errorcluster)  [unwired: 8 in]
        n213 = case shown="True" w516 {
          tunnel: w536 -> [w544 w556]
          tunnel: [w544 w555] -> w535
          tunnel: w534 -> [w546 w554]
          tunnel: [w546 w553] -> w533
          tunnel: [w545 w552] -> w532
          tunnel: [w540 w551] -> w531
          tunnel: w530 -> [w545 w550]
          tunnel: w507 -> [w543 _]
          tunnel: [w539 w547] -> w505
          tunnel: w506 -> [w539 w548]
          tunnel: w504 -> [_ w549]
          frame False {
            (unwired) "Finalization_NG_unit"
            n214 = Select(t="BOOST_MODE", s=w543, f="Finalization_NG_unit") -> (s? t:f=w540:string)
          }
          frame True {
            n215 = call "3.1.1_ECO_Power_Tune.vi"("Data in"=w548, "error in (no error)"=w556, "AllControls In"=w549, 10:w550, "Message Queue out"=w554) -> ("error out"=w555:errorcluster, "Flow"=w551:string, "Data"=w552:T3, "Message Queue Out"=w553:T4, "Data out"=w547:T2)  [unwired: 2 in]
          }
        }
        n216 = Select(t="Enable" ("元素"), s=w516, f="Disable" ("元素")) -> (s? t:f=w515:string)
        n217 = call "Select_Table_Vaule.vi"("Vaule"=w515, "Action"=w519, "Table"=w520) -> ("Result"=w528:bool, "vaule"=w527:string[])  [unwired: 7 in]
        n218 = Append True/False String(1:w528, 2:"FAIL" ("真字符串"), 3:"PASS" ("真字符串")) -> (0:w526:string)  [unwired: 1 in]
        n219 = Build Array (concatenate)(w527, w515, w526) -> (w524:string[])
        n220 = Flush Queue(queue=w533) -> (queue out=w514:T4)  [unwired: 1 in, 2 out]
        n221 = Flatten To XML(anything=w524) -> (xml string=w525:string)
        n222 = call "AMC Send Local Message.vi"("Process (\"\" - local)"=w521, "Message Value"=w525, "Message Name"=w521) -> ()  [unwired: 7 in, 2 out]
      }
    }
    n223 = call "6-AlarmStatus.vi"("Step"=enum16{"Initial", "Write", "Read"}."Read") -> ("AlarmValue Out"=w18:bool[])  [unwired: 9 in, 1 out]
    n224 = call "Stop.vi"("Step"=enum16{"Initial", "Write", "Read"}."Read") -> ("Stop Out"=w26:bool)  [unwired: 9 in, 1 out]
    n225 = call "Exit.vi"("Step"=enum16{"Initial", "Write", "Read"}."Read" ("step")) -> ("Exit Out"=w25:bool)  [unwired: 9 in, 1 out]
    n226 = Or Array Elements(Boolean array=w18) -> (logical OR=w17:bool)
    n227 = Compound Arithmetic op=OR(w24, w26, w25, w17) -> (w23:bool)
    n228 = call "AMC Run Step.vi"("Message Queue In"=w44, "Message Name"=w32, "Message Value"=w30, "error in (no error)"=w39, "Mli/Sig"=FALSE) -> ("Message Queue Out"=w43:T4, "error out"=w38:errorcluster)  [unwired: 13 in]
  }
  "Message Queue Out" <- w6
  "error out" <- w5
  "Data" <- w10
  "Flow" <- w7
  "Data out" <- w2
